vi "Parse Downlink.vi"(7 "CP_DATA IN":u8[](array[numeric]), 8 "error in (no error)":errorcluster, 9 "Parameters":string, 10 "EXID":u32 step=1 format="%06x", 11 "Command":T1) -> (0 "error out":errorcluster, 2 "Downlink":u8[][](array[numeric]) format="%02x")   [LabVIEW 2020]
uses:
  Typedef Command List.ctl
  <vilib>/Utility/miscctls.llb/LVDateTimeRec.ctl
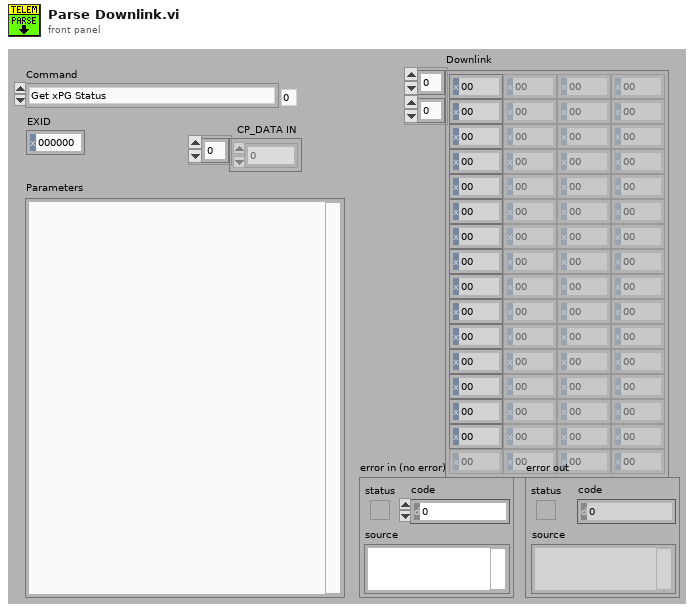
[diagram p1: front panel]
types:
  T1 = typedef "Typedef Command List.ctl" = enum16{"Get xPG Status", "xPG Stimulation", "Select Program", "Increment Program Amplitude", "Decrement Program Amplitude", "Get PoP Constants", "Get PPC Constants", "Get Program Names", "Set Pulse Amplitude", "Increment Pulse Amplitude", "Decrement Pulse Amplitude", "Get Pulse Widths", "Set Pulse Widths", "Increment Pulse Width", "Decrement Pulse Width", "Get Program Frequency", "Set Program Frequency", "Increment Program Frequency", "Decrement Program Frequency", "Inject Event", "Charging Control", "Get xPG Identity", "Set xPG Identity", "Restore Program Defaults", "Get Program Definition", "Set Program Definition", "Get Program Constants", "Set Program Constants", "Get Configurable Device Parameters", "Set Configurable Device Parameters", "Get Pulse Constants", "Set Pulse Constants", "Get Lead Limits", "Set Lead Limits", "Get Channel Calibrations", "Set Channel Calibrations", "<reserved 2>", "<reserved 3>", "<reserved 4>", "<reserved 5>", "<reserved 6>", "<reserved 7>", "Get Stim Asic HV Calibrations", "Set Stim Asic HV Calibrations", "<reserved 8>", "<reserved 9>", "Get CP Data", "Set CP Data", "Clear Log", "Read Log", "Append Log", "Get Patient Program Runtime", "Set Patient Program Runtime", "Impedance Measurement", "Enter Storage Mode", "Echo Short", "Echo Long", "Get General Calibration", "Set General Calibration", "Get Trim List", "Set Trim List", "Get Counter", "Set Counter", "Get Test Stimulation", "Set Test Stimulation", "Get Titration Stimulation", "Set Titration Stimulation", "Get Ramp Time", "Set Ramp Time", "Get VBAT", "Set Software Description Block", "Get Software Description Block", "Write Memory", "Read Memory", "Reset xPG", "Erase Flash Block", "Write Vectors", "Read Vectors", "Diagnostic Data", "Set Background Impedance", "Get Background Impedence ", "Set Test Waveform", "Calibrate Channel", "Get Log Range", "Reserved 0x55", "Reserved 0x56", "MICS Options", "Pair PPC", "Pair POP", "Stop Bootloader", "Tune MICS", "MICS Diagnostics", "Undefined"}
  T2 = enum16{"U8", "U16", "U32", "U64", "I8", "I16", "I32", "I64"}
  T3 = typedef "LVDateTimeRec.ctl" = cluster{"fractional second":dbl, "second":i32, "minute":i32, "hour":i32, "day of month":i32, "month":i32, "year":i32, "day of week":i32, "day of year":i32, "DST":i32}
  T4 = cluster{"CP_DATA IN[0]":u8, "CP_DATA IN[1]":u8, "CP_DATA IN[2]":u8, "CP_DATA IN[3]":u8, "CP_DATA IN[4]":u8, "CP_DATA IN[5]":u8, "CP_DATA IN[6]":u8, "CP_DATA IN[7]":u8, "CP_DATA IN[8]":u8, "CP_DATA IN[9]":u8, "CP_DATA IN[10]":u8, "CP_DATA IN[11]":u8, "CP_DATA IN[12]":u8, "CP_DATA IN[13]":u8, "CP_DATA IN[14]":u8, "CP_DATA IN[15]":u8, "CP_DATA IN[16]":u8, "CP_DATA IN[17]":u8, "CP_DATA IN[18]":u8, "CP_DATA IN[19]":u8, "CP_DATA IN[20]":u8, "CP_DATA IN[21]":u8, "CP_DATA IN[22]":u8, "CP_DATA IN[23]":u8, "CP_DATA IN[24]":u8, "CP_DATA IN[25]":u8, "CP_DATA IN[26]":u8, "CP_DATA IN[27]":u8, "CP_DATA IN[28]":u8, "CP_DATA IN[29]":u8, "CP_DATA IN[30]":u8, "CP_DATA IN[31]":u8, "CP_DATA IN[32]":u8, "CP_DATA IN[33]":u8, "CP_DATA IN[34]":u8, "CP_DATA IN[35]":u8, "CP_DATA IN[36]":u8, "CP_DATA IN[37]":u8, "CP_DATA IN[38]":u8, "CP_DATA IN[39]":u8, "CP_DATA IN[40]":u8, "CP_DATA IN[41]":u8, "CP_DATA IN[42]":u8, "CP_DATA IN[43]":u8, "CP_DATA IN[44]":u8, "CP_DATA IN[45]":u8, "CP_DATA IN[46]":u8, "CP_DATA IN[47]":u8, "CP_DATA IN[48]":u8, "CP_DATA IN[49]":u8, "CP_DATA IN[50]":u8, "CP_DATA IN[51]":u8, "CP_DATA IN[52]":u8, "CP_DATA IN[53]":u8, "CP_DATA IN[54]":u8, "CP_DATA IN[55]":u8, "CP_DATA IN[56]":u8, "CP_DATA IN[57]":u8, "CP_DATA IN[58]":u8, "CP_DATA IN[59]":u8, "CP_DATA IN[60]":u8, "CP_DATA IN[61]":u8, "CP_DATA IN[62]":u8, "CP_DATA IN[63]":u8, "CP_DATA IN[64]":u8, "CP_DATA IN[65]":u8, "CP_DATA IN[66]":u8, "CP_DATA IN[67]":u8, "CP_DATA IN[68]":u8, "CP_DATA IN[69]":u8, "CP_DATA IN[70]":u8, "CP_DATA IN[71]":u8, "CP_DATA IN[72]":u8, "CP_DATA IN[73]":u8, "CP_DATA IN[74]":u8, "CP_DATA IN[75]":u8, "CP_DATA IN[76]":u8, "CP_DATA IN[77]":u8, "CP_DATA IN[78]":u8, "CP_DATA IN[79]":u8, "CP_DATA IN[80]":u8, "CP_DATA IN[81]":u8, "CP_DATA IN[82]":u8, "CP_DATA IN[83]":u8, "CP_DATA IN[84]":u8, "CP_DATA IN[85]":u8, "CP_DATA IN[86]":u8, "CP_DATA IN[87]":u8, "CP_DATA IN[88]":u8, "CP_DATA IN[89]":u8, "CP_DATA IN[90]":u8, "CP_DATA IN[91]":u8, "CP_DATA IN[92]":u8, "CP_DATA IN[93]":u8, "CP_DATA IN[94]":u8, "CP_DATA IN[95]":u8, "CP_DATA IN[96]":u8, "CP_DATA IN[97]":u8, "CP_DATA IN[98]":u8, "CP_DATA IN[99]":u8, "CP_DATA IN[100]":u8, "CP_DATA IN[101]":u8, "CP_DATA IN[102]":u8, "CP_DATA IN[103]":u8, "CP_DATA IN[104]":u8, "CP_DATA IN[105]":u8, "CP_DATA IN[106]":u8, "CP_DATA IN[107]":u8, "CP_DATA IN[108]":u8, "CP_DATA IN[109]":u8, "CP_DATA IN[110]":u8, "CP_DATA IN[111]":u8, "CP_DATA IN[112]":u8, "CP_DATA IN[113]":u8, "CP_DATA IN[114]":u8, "CP_DATA IN[115]":u8, "CP_DATA IN[116]":u8, "CP_DATA IN[117]":u8, "CP_DATA IN[118]":u8, "CP_DATA IN[119]":u8, "CP_DATA IN[120]":u8, "CP_DATA IN[121]":u8, "CP_DATA IN[122]":u8, "CP_DATA IN[123]":u8, "CP_DATA IN[124]":u8, "CP_DATA IN[125]":u8, "CP_DATA IN[126]":u8, "CP_DATA IN[127]":u8, "CP_DATA IN[128]":u8, "CP_DATA IN[129]":u8, "CP_DATA IN[130]":u8, "CP_DATA IN[131]":u8, "CP_DATA IN[132]":u8, "CP_DATA IN[133]":u8, "CP_DATA IN[134]":u8, "CP_DATA IN[135]":u8, "CP_DATA IN[136]":u8, "CP_DATA IN[137]":u8, "CP_DATA IN[138]":u8, "CP_DATA IN[139]":u8, "CP_DATA IN[140]":u8, "CP_DATA IN[141]":u8, "CP_DATA IN[142]":u8, "CP_DATA IN[143]":u8, "CP_DATA IN[144]":u8, "CP_DATA IN[145]":u8, "CP_DATA IN[146]":u8, "CP_DATA IN[147]":u8, "CP_DATA IN[148]":u8, "CP_DATA IN[149]":u8, "CP_DATA IN[150]":u8, "CP_DATA IN[151]":u8, "CP_DATA IN[152]":u8, "CP_DATA IN[153]":u8, "CP_DATA IN[154]":u8, "CP_DATA IN[155]":u8, "CP_DATA IN[156]":u8, "CP_DATA IN[157]":u8, "CP_DATA IN[158]":u8, "CP_DATA IN[159]":u8, "CP_DATA IN[160]":u8, "CP_DATA IN[161]":u8, "CP_DATA IN[162]":u8, "CP_DATA IN[163]":u8, "CP_DATA IN[164]":u8, "CP_DATA IN[165]":u8, "CP_DATA IN[166]":u8, "CP_DATA IN[167]":u8, "CP_DATA IN[168]":u8, "CP_DATA IN[169]":u8, "CP_DATA IN[170]":u8, "CP_DATA IN[171]":u8, "CP_DATA IN[172]":u8, "CP_DATA IN[173]":u8, "CP_DATA IN[174]":u8, "CP_DATA IN[175]":u8, "CP_DATA IN[176]":u8, "CP_DATA IN[177]":u8, "CP_DATA IN[178]":u8, "CP_DATA IN[179]":u8, "CP_DATA IN[180]":u8, "CP_DATA IN[181]":u8, "CP_DATA IN[182]":u8, "CP_DATA IN[183]":u8, "CP_DATA IN[184]":u8, "CP_DATA IN[185]":u8, "CP_DATA IN[186]":u8, "CP_DATA IN[187]":u8, "CP_DATA IN[188]":u8, "CP_DATA IN[189]":u8, "CP_DATA IN[190]":u8, "CP_DATA IN[191]":u8, "CP_DATA IN[192]":u8, "CP_DATA IN[193]":u8, "CP_DATA IN[194]":u8, "CP_DATA IN[195]":u8, "CP_DATA IN[196]":u8, "CP_DATA IN[197]":u8, "CP_DATA IN[198]":u8, "CP_DATA IN[199]":u8, "CP_DATA IN[200]":u8, "CP_DATA IN[201]":u8, "CP_DATA IN[202]":u8, "CP_DATA IN[203]":u8, "CP_DATA IN[204]":u8, "CP_DATA IN[205]":u8, "CP_DATA IN[206]":u8, "CP_DATA IN[207]":u8, "CP_DATA IN[208]":u8, "CP_DATA IN[209]":u8, "CP_DATA IN[210]":u8, "CP_DATA IN[211]":u8, "CP_DATA IN[212]":u8, "CP_DATA IN[213]":u8, "CP_DATA IN[214]":u8, "CP_DATA IN[215]":u8, "CP_DATA IN[216]":u8, "CP_DATA IN[217]":u8, "CP_DATA IN[218]":u8, "CP_DATA IN[219]":u8, "CP_DATA IN[220]":u8, "CP_DATA IN[221]":u8, "CP_DATA IN[222]":u8, "CP_DATA IN[223]":u8, "CP_DATA IN[224]":u8, "CP_DATA IN[225]":u8, "CP_DATA IN[226]":u8, "CP_DATA IN[227]":u8, "CP_DATA IN[228]":u8, "CP_DATA IN[229]":u8, "CP_DATA IN[230]":u8, "CP_DATA IN[231]":u8, "CP_DATA IN[232]":u8, "CP_DATA IN[233]":u8, "CP_DATA IN[234]":u8, "CP_DATA IN[235]":u8, "CP_DATA IN[236]":u8, "CP_DATA IN[237]":u8, "CP_DATA IN[238]":u8, "CP_DATA IN[239]":u8, "CP_DATA IN[240]":u8, "CP_DATA IN[241]":u8, "CP_DATA IN[242]":u8, "CP_DATA IN[243]":u8, "CP_DATA IN[244]":u8, "CP_DATA IN[245]":u8, "CP_DATA IN[246]":u8, "CP_DATA IN[247]":u8, "CP_DATA IN[248]":u8, "CP_DATA IN[249]":u8, "CP_DATA IN[250]":u8, "CP_DATA IN[251]":u8, "CP_DATA IN[252]":u8, "CP_DATA IN[253]":u8, "CP_DATA IN[254]":u8, "CP_DATA IN[255]":u8}
  T5 = cluster{"DATA[0]":u8, "DATA[1]":u8, "DATA[2]":u8, "DATA[3]":u8, "DATA[4]":u8, "DATA[5]":u8, "DATA[6]":u8, "DATA[7]":u8, "DATA[8]":u8, "DATA[9]":u8, "DATA[10]":u8, "DATA[11]":u8, "DATA[12]":u8, "DATA[13]":u8, "DATA[14]":u8}
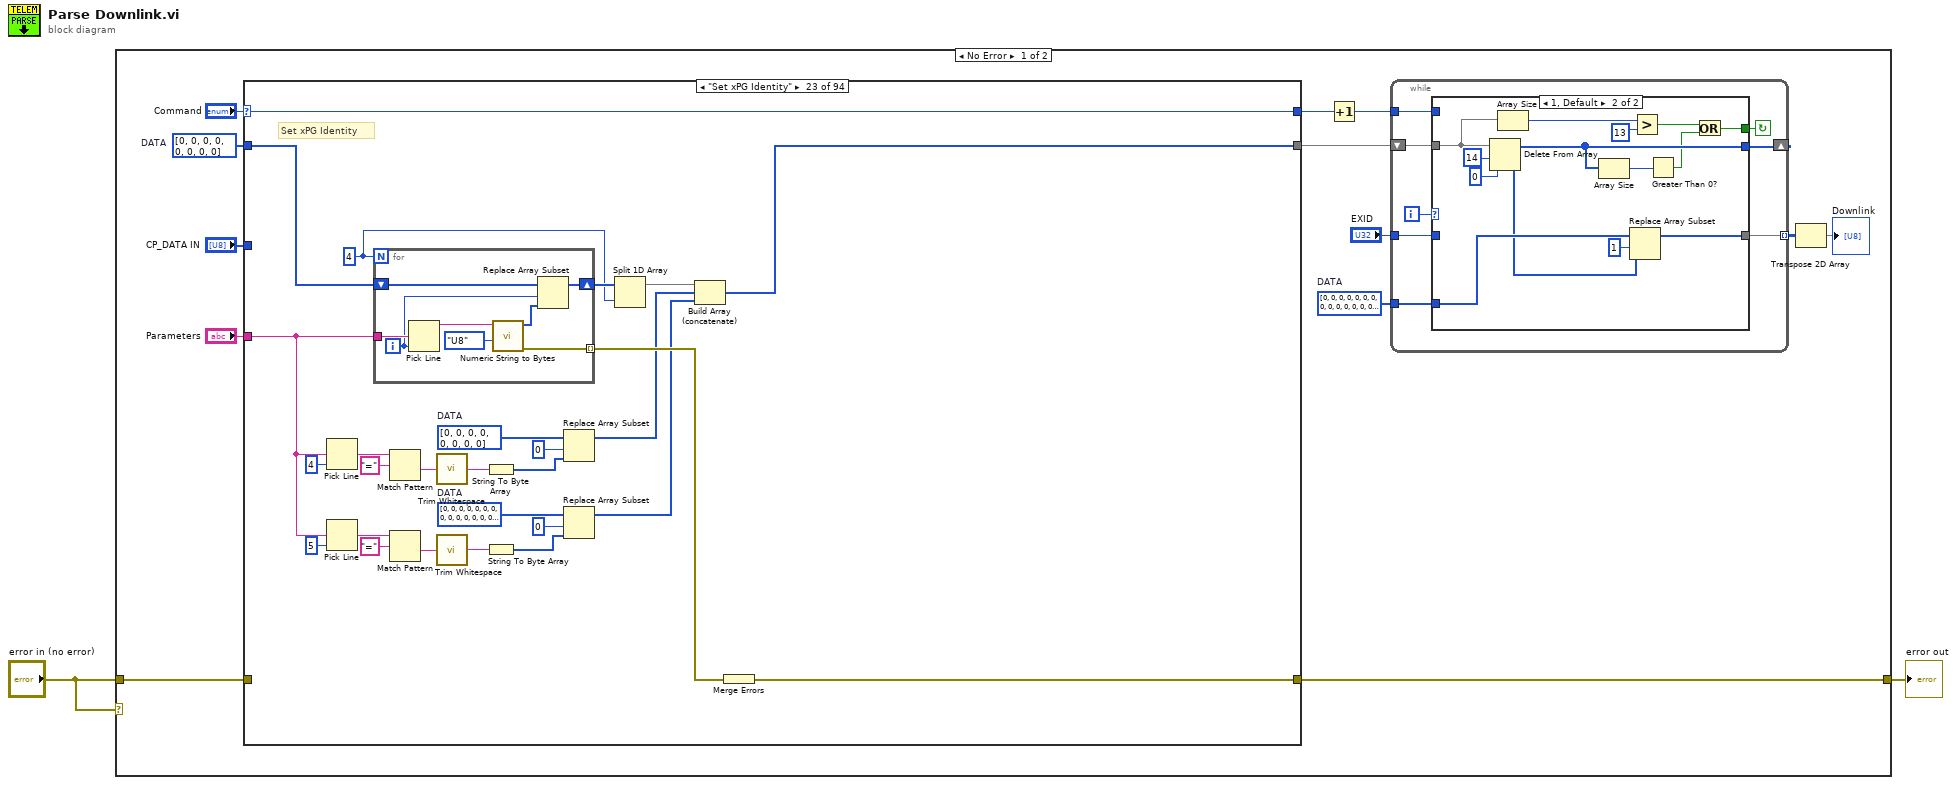
[diagram p0: block diagram]
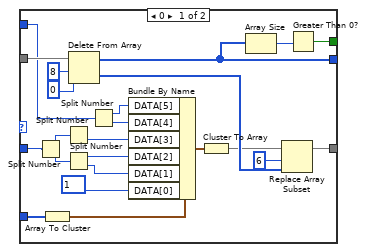
[diagram p2: hidden frame]
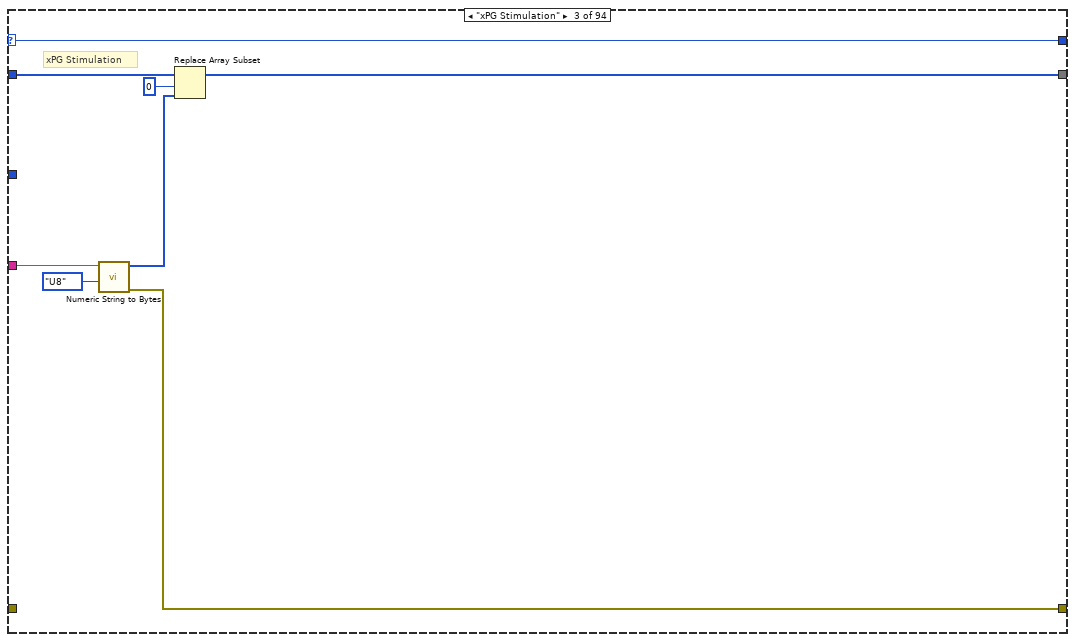
[diagram p5: hidden frame]
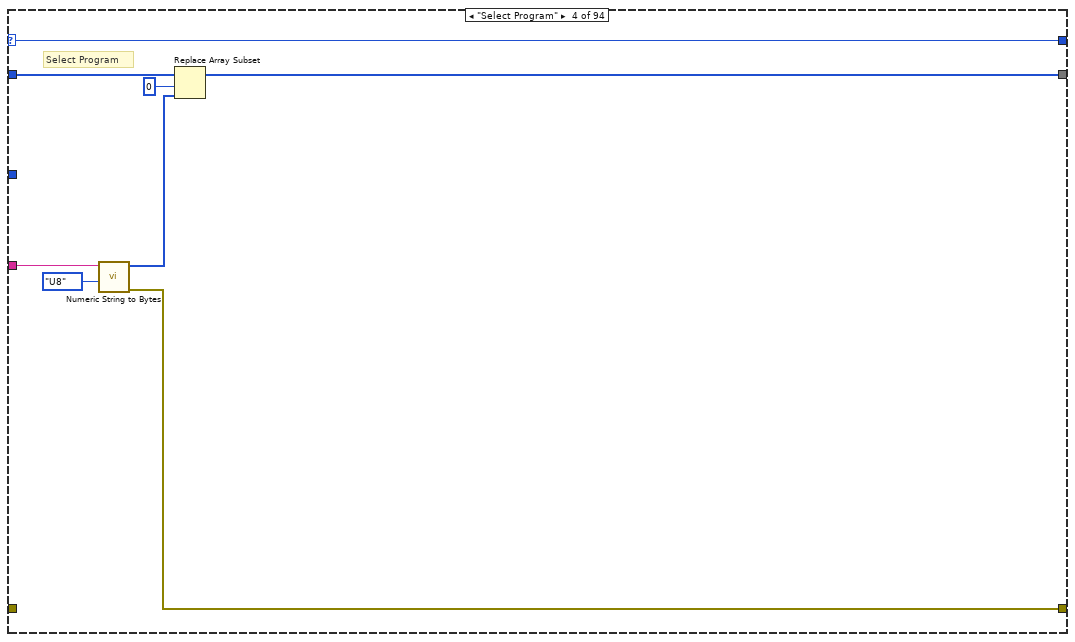
[diagram p6: hidden frame]
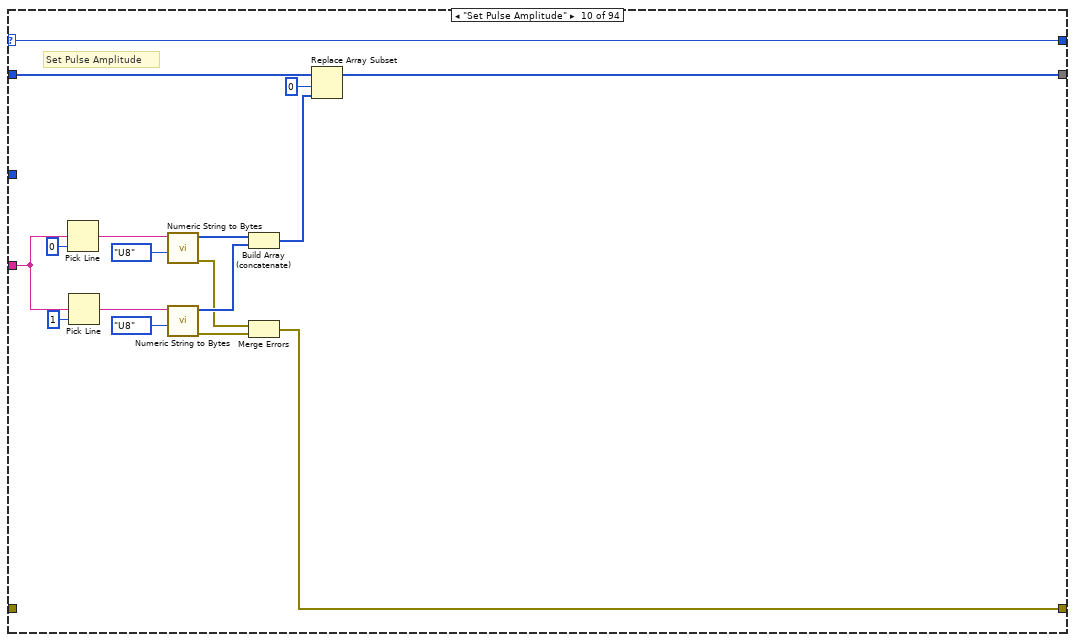
[diagram p12: hidden frame]
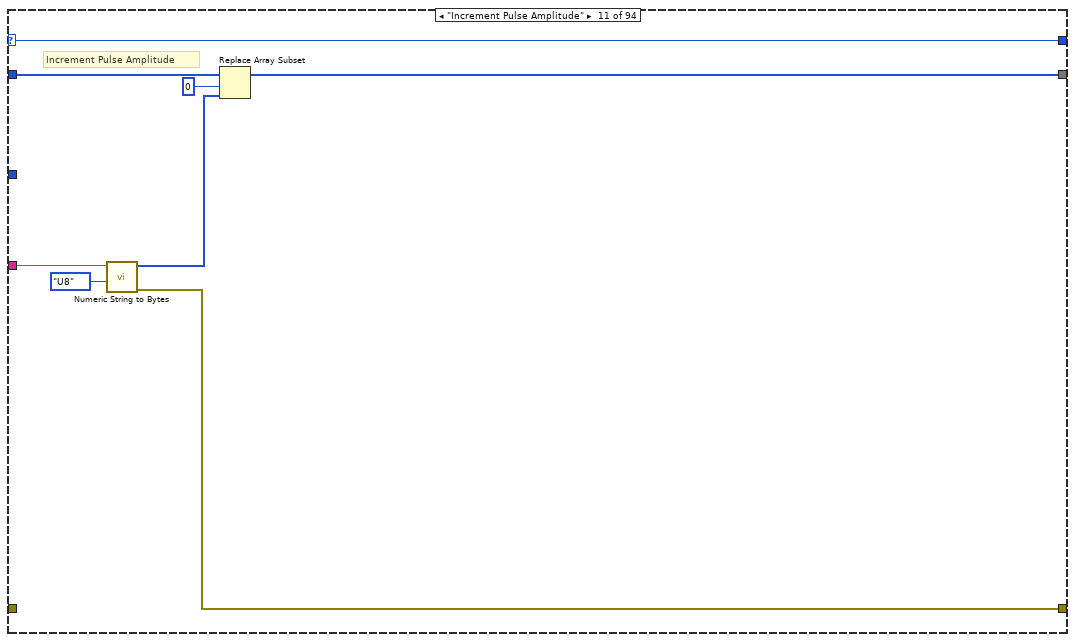
[diagram p13: hidden frame]
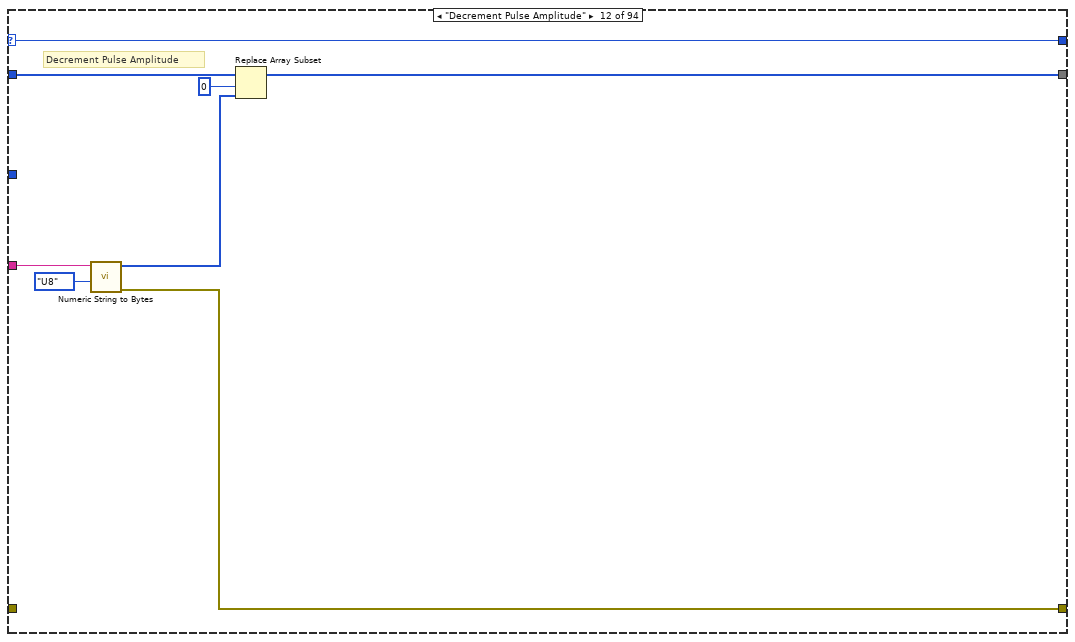
[diagram p14: hidden frame]
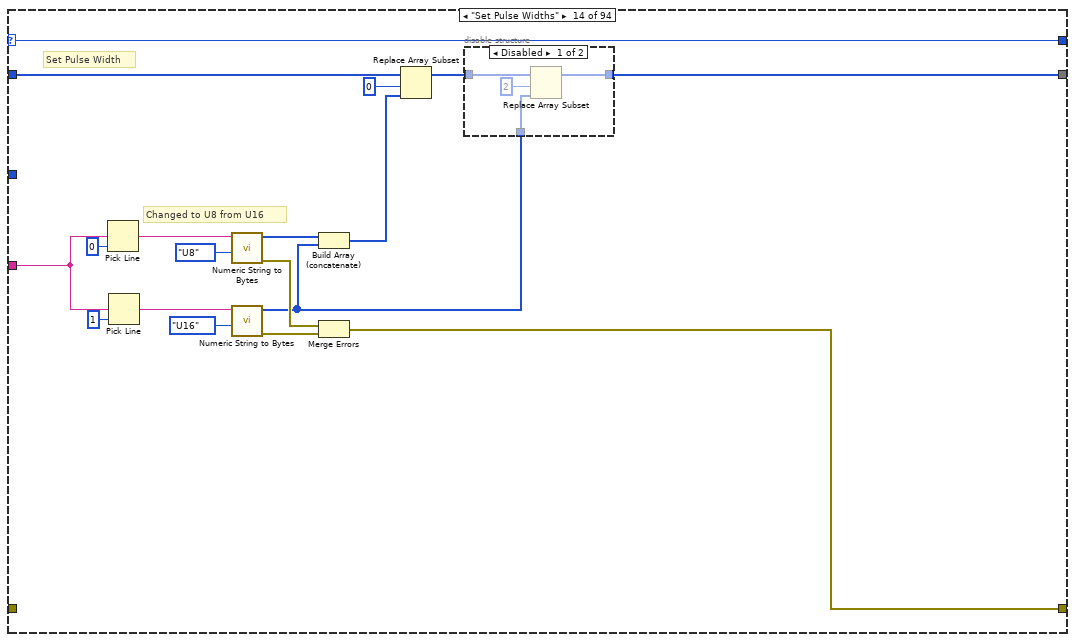
[diagram p16: hidden frame]
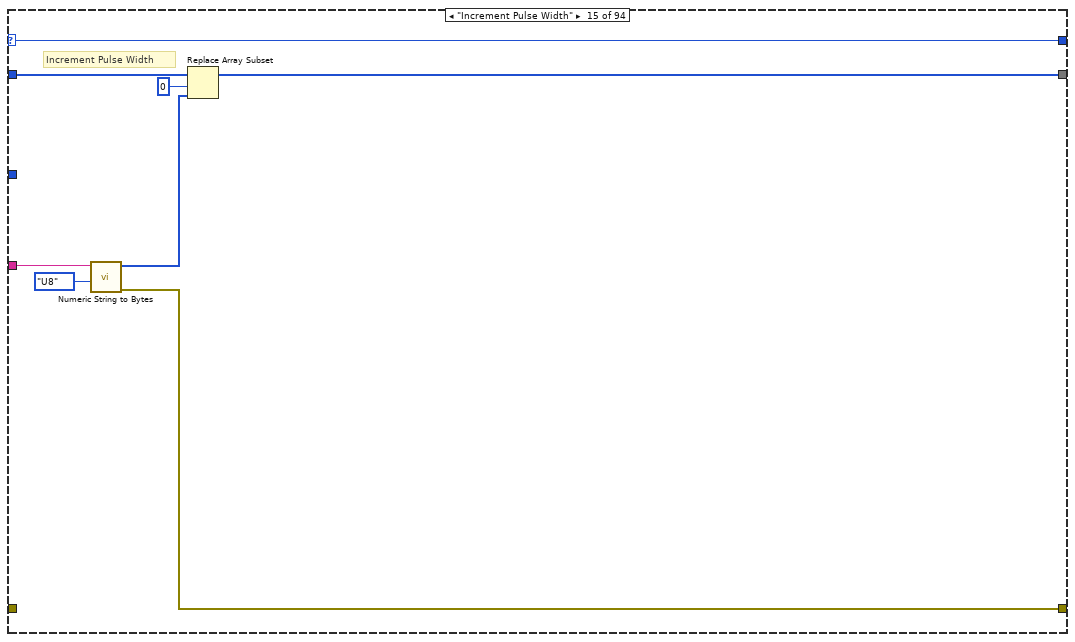
[diagram p18: hidden frame]
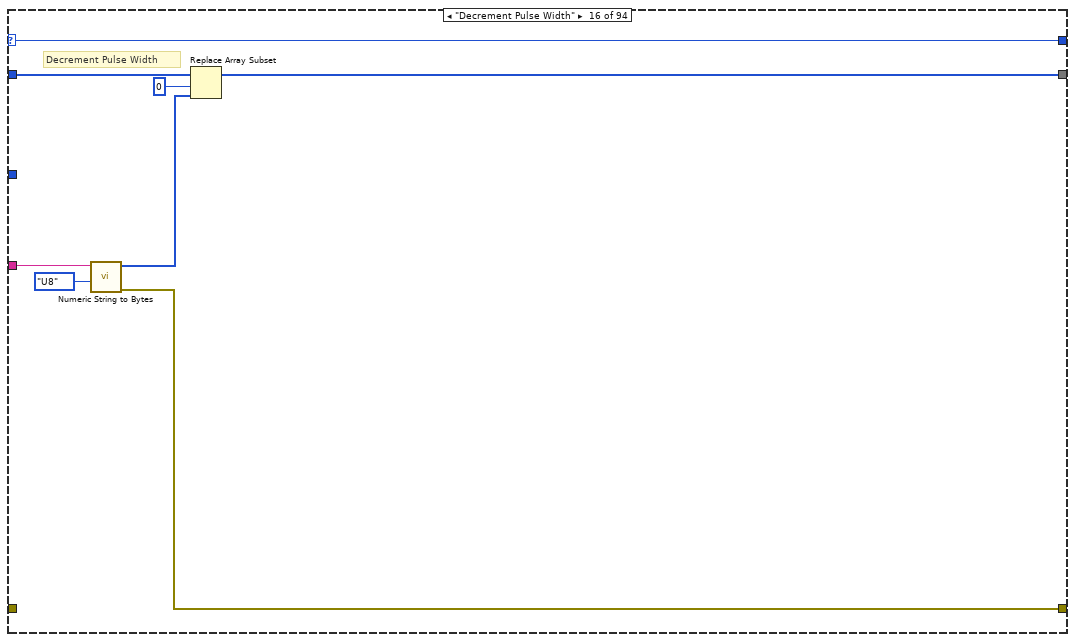
[diagram p19: hidden frame]
diagram:
  n1 = case shown="No Error" "error in (no error)" {
    tunnel: "error in (no error)" -> [w8 w1324]
    tunnel: [w7 w1324] -> w2
    frame No Error {
      w9 = u8[] [0, 0, 0, 0, 0, 0, 0, 0]  # DATA
      w10 = u8[] [0, 0, 0, 0, 0, 0, 0, 0, 0, 0, 0, 0, 0, 0, 0]  # DATA
      n2 = case shown="\"Set xPG Identity\"" "Command" {
        selector: "Command" -> [w63 w66 w74 w82 w85 w88 w91 w94 w97 w114 w122 w130 w133 w151 w164 w172 w175 w183 w186 w189 w192 w195 w222 w238 w246 w253 w396 w410 w423 w498 w516 w535 w546 w553 w569 w582 w594 w601 w617 w629 w637 w656 w694 w702 w720 w743 w746 w752 w758 w761 w767 w869 w871 w961 w980 w983 w1007 w1064 w1083 w1115 w1123 w1126 w1129 w1132 w1154 w1171 w1174 w1177 w1180 w1183 w1200 w1214 w1228 w1231 w1233 w1236 w1247 w1249 w1252 w1255 w1258 w1261 w1264 w1267 w1296 w1298 w1301 w1304 w1307 w1310 w1313 w1316 w1319 w1322]
        tunnel: "Parameters" -> [_ _ w72 w80 _ _ _ _ _ w113 w120 w128 _ w139 w162 w170 _ w181 _ _ _ _ w221 w236 w244 w248 _ w398 _ w428 _ w522 _ w550 w564 w571 _ w598 w615 w624 w635 w640 w659 w700 w703 w721 _ _ _ _ w763 w864 w873 w959 w964 _ w989 _ w1074 _ w1120 _ _ _ w1143 w1166 _ _ _ _ w1196 w1204 w1218 _ _ _ w1245 _ _ _ _ _ _ _ w1287 _ _ _ _ _ _ _ _ _]
        tunnel: [w63 w66 w74 w82 w85 w88 w91 w94 w97 w114 w122 w130 w133 w151 w164 w172 w175 w183 w186 w189 w192 w195 w222 w238 w246 w253 w396 w410 w423 w498 w516 w535 w546 w553 w569 w582 w594 w601 w617 w629 w637 w656 w694 w702 w720 w743 w746 w752 w758 w761 w767 w869 w871 w961 w980 w983 w1007 w1064 w1083 w1115 w1123 w1126 w1129 w1132 w1154 w1171 w1174 w1177 w1180 w1183 w1200 w1214 w1228 w1231 w1233 w1236 w1247 w1249 w1252 w1255 w1258 w1261 w1264 w1267 w1296 w1298 w1301 w1304 w1307 w1310 w1313 w1316 w1319 w1322] -> w15
        tunnel: [w62 w65 w70 w78 w84 w87 w90 w93 w96 w106 w118 w126 w132 w137 w160 w168 w174 w179 w185 w188 w191 w194 w201 w234 w242 w249 w395 w408 w422 w495 w515 w532 w545 w548 w562 w574 w593 w596 w613 w623 w633 w654 w692 w698 w718 w741 w745 w748 w754 w760 w764 w862 w872 w957 w978 w981 w986 w1062 w1069 w1113 w1117 w1124 w1127 w1130 w1142 w1155 w1172 w1175 w1178 w1181 w1184 w1209 w1223 w1230 w1232 w1235 w1239 w1248 w1251 w1254 w1257 w1260 w1263 w1266 w1271 w1297 w1300 w1303 w1306 w1309 w1312 w1315 w1318 w1321] -> w13
        tunnel: w9 -> [w62 w65 w73 w81 w84 w87 w90 w93 w96 w105 w121 w129 w132 w144 w163 w171 w174 w182 w185 w188 w191 w194 w212 w237 w245 _ w395 _ w422 _ w515 _ w545 _ w563 _ w593 _ w616 _ w636 w655 w693 w701 w719 w742 w745 _ _ w760 _ w865 _ w960 w979 w981 _ w1062 _ w1113 w1119 w1124 w1127 w1130 _ w1156 w1172 w1175 w1178 w1181 w1187 _ _ w1230 w1232 w1235 w1241 w1248 w1251 w1254 w1257 w1260 w1263 w1266 w1272 w1297 w1300 w1303 w1306 w1309 w1312 w1315 w1318 w1321]
        tunnel: w8 -> [w61 w64 _ _ w83 w86 w89 w92 w95 _ _ _ w131 _ _ _ w173 _ w184 w187 w190 w193 _ _ _ w251 w394 _ w421 _ w514 _ w544 _ _ _ w592 _ _ _ _ _ _ _ _ _ w744 w747 w753 w759 _ _ _ _ _ w982 _ w1063 _ w1114 _ w1125 w1128 w1131 _ _ w1173 w1176 w1179 w1182 _ _ _ w1229 w1234 w1237 _ w1250 w1253 w1256 w1259 w1262 w1265 w1268 _ w1299 w1302 w1305 w1308 w1311 w1314 w1317 w1320 w1323]
        tunnel: [w61 w64 w71 w79 w83 w86 w89 w92 w95 w98 w119 w127 w131 w140 w161 w169 w173 w180 w184 w187 w190 w193 w202 w235 w243 w250 w394 w401 w421 w496 w514 w531 w544 w551 w565 w580 w592 w599 w614 w628 w634 w641 w678 w699 w704 w727 w744 w747 w753 w759 w765 w863 w870 w958 w965 w982 w987 w1063 w1065 w1114 w1116 w1125 w1128 w1131 w1141 w1157 w1173 w1176 w1179 w1182 w1188 w1201 w1215 w1229 w1234 w1237 w1238 w1250 w1253 w1256 w1259 w1262 w1265 w1268 w1274 w1299 w1302 w1305 w1308 w1311 w1314 w1317 w1320 w1323] -> w7
        tunnel: "CP_DATA IN" -> [_ _ _ _ _ _ _ _ _ _ _ _ _ _ _ _ _ _ _ _ _ _ _ _ _ _ _ _ _ _ _ _ _ _ _ _ _ _ _ w620 _ _ _ _ _ _ _ w751 w757 _ _ _ _ _ _ _ _ _ _ _ _ _ _ _ w1134 _ _ _ _ _ _ _ _ _ _ _ _ _ _ _ _ _ _ _ _ _ _ _ _ _ _ _ _ _]
        frame Default {
          # "NULL"
        }
        frame "Get xPG Status" {
          # "Get xPG Status"
        }
        frame "xPG Stimulation" {
          # "xPG Stimulation"
          n3 = call "Numeric String to Bytes.vi"("Type"=T2."U8", "String"=w72) -> ("error out"=w71:errorcluster, "Byte Data"=w68:u8[])  [unwired: 8 in]
          n4 = Replace Array Subset(array=w73, new element=w68, index=0) -> (w70:u8[])
        }
        frame "Select Program" {
          # "Select Program"
          n5 = call "Numeric String to Bytes.vi"("Type"=T2."U8", "String"=w80) -> ("error out"=w79:errorcluster, "Byte Data"=w76:u8[])  [unwired: 8 in]
          n6 = Replace Array Subset(array=w81, new element=w76, index=0) -> (w78:u8[])
        }
        frame "Increment Program Amplitude" {
          # "Increment Program Amplitude"
        }
        frame "Decrement Program Amplitude" {
          # "Decrement Program Amplitude"
        }
        frame "Get PoP Constants" {
          # "Get PoP Constants"
        }
        frame "Get PPC Constants" {
          # "Get PPC Constants"
        }
        frame "Get Program Names" {
          # "Get Program Names"
        }
        frame "Set Pulse Amplitude" {
          # "Set Pulse Amplitude"
          n7 = Pick Line(multi-line string=w113, line index=0) -> (output string=w107:string)  [unwired: 1 in]
          n8 = Pick Line(multi-line string=w113, line index=1) -> (output string=w108:string)  [unwired: 1 in]
          n9 = call "Numeric String to Bytes.vi"("Type"=T2."U8", "String"=w107) -> ("error out"=w100:errorcluster, "Byte Data"=w104:u8[])  [unwired: 8 in]
          n10 = call "Numeric String to Bytes.vi"("Type"=T2."U8", "String"=w108) -> ("error out"=w99:errorcluster, "Byte Data"=w103:u8[])  [unwired: 8 in]
          n11 = Build Array (concatenate)(w104, w103) -> (w101:u8[])
          n12 = Merge Errors(w100, w99) -> (w98:errorcluster)
          n13 = Replace Array Subset(array=w105, new element=w101, index=0) -> (w106:u8[])
        }
        frame "Increment Pulse Amplitude" {
          # "Increment Pulse Amplitude"
          n14 = call "Numeric String to Bytes.vi"("Type"=T2."U8", "String"=w120) -> ("error out"=w119:errorcluster, "Byte Data"=w116:u8[])  [unwired: 8 in]
          n15 = Replace Array Subset(array=w121, new element=w116, index=0) -> (w118:u8[])
        }
        frame "Decrement Pulse Amplitude" {
          # "Decrement Pulse Amplitude"
          n16 = call "Numeric String to Bytes.vi"("Type"=T2."U8", "String"=w128) -> ("error out"=w127:errorcluster, "Byte Data"=w124:u8[])  [unwired: 8 in]
          n17 = Replace Array Subset(array=w129, new element=w124, index=0) -> (w126:u8[])
        }
        frame "Get Pulse Widths" {
          # "Get Pulse Widths"
        }
        frame "Set Pulse Widths" {
          # "Changed to U8 from U16"
          # "Set Pulse Width"
          n18 = Pick Line(multi-line string=w139, line index=0) -> (output string=w145:string)  [unwired: 1 in]
          n19 = Pick Line(multi-line string=w139, line index=1) -> (output string=w146:string)  [unwired: 1 in]
          n20 = call "Numeric String to Bytes.vi"("Type"=T2."U8", "String"=w145) -> ("error out"=w142:errorcluster, "Byte Data"=w136:u8[])  [unwired: 8 in]
          n21 = call "Numeric String to Bytes.vi"("Type"=T2."U16", "String"=w146) -> ("error out"=w141:errorcluster, "Byte Data"=w135:u8[])  [unwired: 8 in]
          n22 = Build Array (concatenate)(w136, w135) -> (w134:u8[])
          n23 = Merge Errors(w142, w141) -> (w140:errorcluster)
          n24 = Replace Array Subset(array=w144, new element=w134, index=0) -> (w138:u8[])
          n25 = disable-structure shown="Disabled" {
            disable-tunnel: w135 -> [w154 _]
            disable-tunnel: w138 -> [w153 w156]
            disable-tunnel: [w152 w156] -> w137
            frame Disabled {
              n26 = Replace Array Subset(array=w153, new element=w154, index=2) -> (w152:u8[])
            }
            frame Enabled {
            }
          }
        }
        frame "Increment Pulse Width" {
          # "Increment Pulse Width"
          n27 = call "Numeric String to Bytes.vi"("Type"=T2."U8", "String"=w162) -> ("error out"=w161:errorcluster, "Byte Data"=w158:u8[])  [unwired: 8 in]
          n28 = Replace Array Subset(array=w163, new element=w158, index=0) -> (w160:u8[])
        }
        frame "Decrement Pulse Width" {
          # "Decrement Pulse Width"
          n29 = call "Numeric String to Bytes.vi"("Type"=T2."U8", "String"=w170) -> ("error out"=w169:errorcluster, "Byte Data"=w166:u8[])  [unwired: 8 in]
          n30 = Replace Array Subset(array=w171, new element=w166, index=0) -> (w168:u8[])
        }
        frame "Get Program Frequency" {
          # "Get Program Frequency"
        }
        frame "Set Program Frequency" {
          # "Set Program Frequency"
          n31 = call "Numeric String to Bytes.vi"("Type"=T2."U8", "String"=w181) -> ("error out"=w180:errorcluster, "Byte Data"=w177:u8[])  [unwired: 8 in]
          n32 = Replace Array Subset(array=w182, new element=w177, index=0) -> (w179:u8[])
        }
        frame "Increment Program Frequency" {
          # "Increment Program Frequency"
        }
        frame "Decrement Program Frequency" {
          # "Decrement Program Frequency"
        }
        frame "Charging Control" {
          # "Charging Control"
        }
        frame "Get xPG Identity" {
          # "Get xPG Identity"
        }
        frame "Set xPG Identity" {
          w215 = u8[] [0, 0, 0, 0, 0, 0, 0, 0, 0, 0, 0, 0, 0, 0, 0, 0]  # DATA
          w216 = u8[] [0, 0, 0, 0, 0, 0, 0, 0]  # DATA
          w199 = 4
          # "Set xPG Identity"
          n33 = Pick Line(multi-line string=w221, line index=4) -> (output string=w208:string)  [unwired: 1 in]
          n34 = Pick Line(multi-line string=w221, line index=5) -> (output string=w205:string)  [unwired: 1 in]
          n35 = for {
            N: w199 -> [_]
            tunnel: w221 -> [w230]
            shift-right: [w225] -> w200
            shift-left: w212 -> [w226]
            tunnel: [w227] -> w203 mode=indexing
            i -> [w223]
            n36 = Pick Line(multi-line string=w230, line index=w223) -> (output string=w229:string)  [unwired: 1 in]
            n37 = call "Numeric String to Bytes.vi"("Type"=T2."U8", "String"=w229) -> ("error out"=w227:errorcluster, "Byte Data"=w224:u8[])  [unwired: 8 in]
            n38 = Replace Array Subset(array=w226, new element=w224, index=w223) -> (w225:u8[])
          }
          n39 = Match Pattern(string=w208, regular expression="=") -> (after substring=w207:string)  [unwired: 1 in, 3 out]
          n40 = Match Pattern(string=w205, regular expression="=") -> (after substring=w204:string)  [unwired: 1 in, 3 out]
          n41 = call <vilib>:"Trim Whitespace.vi"("string"=w207) -> ("trimmed string"=w218:string)  [unwired: 1 in]
          n42 = call <vilib>:"Trim Whitespace.vi"("string"=w204) -> ("trimmed string"=w217:string)  [unwired: 1 in]
          n43 = String To Byte Array(string=w218) -> (unsigned byte array=w213:u8[])
          n44 = String To Byte Array(string=w217) -> (unsigned byte array=w214:u8[])
          n45 = Replace Array Subset(array=w216, new element=w213, index=0) -> (w197:u8[])
          n46 = Replace Array Subset(array=w215, new element=w214, index=0) -> (w196:u8[])
          n47 = Split 1D Array(array=w200, index=w199) -> (first subarray=w198:u8[])  [unwired: 1 out]
          n48 = Build Array (concatenate)(w198, w197, w196) -> (w201:u8[])
          n49 = Merge Errors(w203) -> (w202:errorcluster)
        }
        frame "Restore Program Defaults" {
          # "Restore Program Defaults"
          n50 = call "Numeric String to Bytes.vi"("Type"=T2."U16", "String"=w236) -> ("error out"=w235:errorcluster, "Byte Data"=w232:u8[])  [unwired: 8 in]
          n51 = Replace Array Subset(array=w237, new element=w232, index=0) -> (w234:u8[])
        }
        frame "Get Program Definition" {
          # "Get Program Definition"
          n52 = call "Numeric String to Bytes.vi"("Type"=T2."U8", "String"=w244) -> ("error out"=w243:errorcluster, "Byte Data"=w240:u8[])  [unwired: 8 in]
          n53 = Replace Array Subset(array=w245, new element=w240, index=0) -> (w242:u8[])
        }
        frame "Set Program Definition" {
          w252 = u8[] []  # DATA
          # "Set Program Definition"
          n54 = while {
            shift-right: [w257] -> w249
            shift-left: w252 -> [w258]
            shift-right: [w263] -> w250
            shift-left: w251 -> [w264]
            tunnel: w248 -> [w256]
            shift-right: [w254] -> _
            shift-left: 0 -> [w255]
            i -> [w259]
            stop <- w260 stop-if-true
            n55 = case shown="0" w259 {
              tunnel: w264 -> [w276 w328]
              tunnel: [w275 w327] -> w263
              tunnel: [FALSE ("status") TRUE ("status")] -> w261
              tunnel: w258 -> [w289 w331]
              tunnel: [w288 w330] -> w257
              tunnel: w256 -> [w291 w325]
              tunnel: w255 -> [_ w326]
              tunnel: [14 ("line index") w323] -> w254
              frame 0 {
                w305 = u8[] [0, 0, 0, 0, 0, 0, 0, 0, 0, 0, 0, 0, 0, 0, 0, 0]  # DATA
                # "Changed to U8 from U16"
                n56 = Pick Line(multi-line string=w291, line index=3) -> (output string=w272:string)  [unwired: 1 in]
                n57 = Pick Line(multi-line string=w291, line index=0) -> (output string=w298:string)  [unwired: 1 in]
                n58 = Pick Line(multi-line string=w291, line index=1) -> (output string=w299:string)  [unwired: 1 in]
                n59 = Pick Line(multi-line string=w291, line index=2) -> (output string=w300:string)  [unwired: 1 in]
                n60 = Pick Line(multi-line string=w291, line index=12) -> (output string=w295:string)  [unwired: 1 in]
                n61 = Pick Line(multi-line string=w291, line index=13) -> (output string=w292:string)  [unwired: 1 in]
                n62 = for {
                  N: 8 -> [_]
                  tunnel: w291 -> [w322]
                  shift-right: [w314] -> w285
                  shift-left: w289 -> [w315]
                  tunnel: [w313] -> w270 mode=indexing
                  i -> [w320]
                  n63 = Add(x=4 ("line index"), y=w320) -> (x+y=w319:i32)
                  n64 = Pick Line(multi-line string=w322, line index=w319) -> (output string=w317:string)  [unwired: 1 in]
                  n65 = call "Numeric String to Bytes.vi"("Type"=T2."U8", "String"=w317) -> ("error out"=w313:errorcluster, "Byte Data"=w316:u8[])  [unwired: 8 in]
                  n66 = Build Array (concatenate)(w315, w316) -> (w314:u8[])
                }
                n67 = Match Pattern(string=w272, regular expression="=") -> (after substring=w271:string)  [unwired: 1 in, 3 out]
                n68 = call <vilib>:"Trim Whitespace.vi"("string"=w271) -> ("trimmed string"=w308:string)  [unwired: 1 in]
                n69 = call "Numeric String to Bytes.vi"("Type"=T2."U8", "String"=w298) -> ("error out"=w281:errorcluster, "Byte Data"=w287:u8[])  [unwired: 8 in]
                n70 = call "Numeric String to Bytes.vi"("Type"=T2."U8", "String"=w299) -> ("error out"=w280:errorcluster, "Byte Data"=w269:u8[])  [unwired: 8 in]
                n71 = call "Numeric String to Bytes.vi"("Type"=T2."U8", "String"=w300) -> ("error out"=w279:errorcluster, "Byte Data"=w286:u8[])  [unwired: 8 in]
                n72 = call "Numeric String to Bytes.vi"("Type"=T2."U8", "String"=w295) -> ("error out"=w278:errorcluster, "Byte Data"=w284:u8[])  [unwired: 8 in]
                n73 = call "Numeric String to Bytes.vi"("Type"=T2."U8", "String"=w292) -> ("error out"=w277:errorcluster, "Byte Data"=w283:u8[])  [unwired: 8 in]
                n74 = String To Byte Array(string=w308) -> (unsigned byte array=w307:u8[])
                n75 = Replace Array Subset(array=w305, new element=w307, index=0) -> (w265:u8[])
                n76 = Split 1D Array(array=w265, index=16) -> (first subarray=w266:u8[])  [unwired: 1 out]
                n77 = Build Array (concatenate)(w289, w287, u8[] [0] ("array"), w269, w286, w266, w285, w284, w283) -> (w288:u8[])
                n78 = Build Array (concatenate)(w281, w280, w279, w270, w278, w277, w276) -> (w274:errorcluster[])
                n79 = Merge Errors(w274) -> (w275:errorcluster)
              }
              frame 1, Default {
                n80 = for {
                  N: 4 -> [_]
                  shift-right: [w349] -> w330
                  shift-left: w331 -> [w366]
                  shift-right: [w351] -> w327
                  shift-left: w328 -> [w358]
                  tunnel: w325 -> [w343]
                  shift-right: [w337] -> w323
                  shift-left: w326 -> [w344]
                  w342 = u8[] []  # DATA
                  w335 = u8[] [0, 0, 0, 0, 0, 0, 0, 0, 0, 0, 0, 0, 0, 0, 0, 0]  # DATA
                  n81 = Increment(x=w344) -> (x+1=w338:i32)
                  n82 = Increment(x=w338) -> (x+1=w369:i32)
                  n83 = Pick Line(multi-line string=w343, line index=w344) -> (output string=w341:string)  [unwired: 1 in]
                  n84 = Pick Line(multi-line string=w343, line index=w338) -> (output string=w381:string)  [unwired: 1 in]
                  n85 = Increment(x=w369) -> (x+1=w370:i32)
                  n86 = Pick Line(multi-line string=w343, line index=w369) -> (output string=w382:string)  [unwired: 1 in]
                  n87 = Match Pattern(string=w341, regular expression="=") -> (after substring=w340:string)  [unwired: 1 in, 3 out]
                  n88 = Increment(x=w370) -> (x+1=w371:i32)
                  n89 = Pick Line(multi-line string=w343, line index=w370) -> (output string=w375:string)  [unwired: 1 in]
                  n90 = Increment(x=w371) -> (x+1=w372:i32)
                  n91 = Pick Line(multi-line string=w343, line index=w371) -> (output string=w376:string)  [unwired: 1 in]
                  n92 = call <vilib>:"Trim Whitespace.vi"("string"=w340) -> ("trimmed string"=w347:string)  [unwired: 1 in]
                  n93 = Increment(x=w372) -> (x+1=w368:i32)
                  n94 = Pick Line(multi-line string=w343, line index=w372) -> (output string=w377:string)  [unwired: 1 in]
                  n95 = Increment(x=w368) -> (x+1=w367:i32)
                  n96 = String To Byte Array(string=w347) -> (unsigned byte array=w346:u8[])
                  n97 = Pick Line(multi-line string=w343, line index=w368) -> (output string=w373:string)  [unwired: 1 in]
                  n98 = for {
                    N: 26 -> [_]
                    tunnel: w343 -> [w393]
                    shift-right: [w388] -> w359
                    shift-left: w342 -> [w389]
                    shift-right: [w386] -> w337
                    shift-left: w367 -> [w387]
                    tunnel: [w385] -> w336 mode=indexing
                    n99 = Pick Line(multi-line string=w393, line index=w387) -> (output string=w391:string)  [unwired: 1 in]
                    n100 = Increment(x=w387) -> (x+1=w386:i32)
                    n101 = call "Numeric String to Bytes.vi"("Type"=T2."I8", "String"=w391) -> ("error out"=w385:errorcluster, "Byte Data"=w390:u8[])  [unwired: 8 in]
                    n102 = Build Array (concatenate)(w389, w390) -> (w388:u8[])
                  }
                  n103 = Replace Array Subset(array=w335, new element=w346, index=0) -> (w333:u8[])
                  n104 = call "Numeric String to Bytes.vi"("Type"=T2."U16", "String"=w381) -> ("error out"=w357:errorcluster, "Byte Data"=w365:u8[])  [unwired: 8 in]
                  n105 = call "Numeric String to Bytes.vi"("Type"=T2."U16", "String"=w382) -> ("error out"=w356:errorcluster, "Byte Data"=w364:u8[])  [unwired: 8 in]
                  n106 = call "Numeric String to Bytes.vi"("Type"=T2."I16", "String"=w375) -> ("error out"=w355:errorcluster, "Byte Data"=w363:u8[])  [unwired: 8 in]
                  n107 = call "Numeric String to Bytes.vi"("Type"=T2."U16", "String"=w376) -> ("error out"=w354:errorcluster, "Byte Data"=w362:u8[])  [unwired: 8 in]
                  n108 = call "Numeric String to Bytes.vi"("Type"=T2."U16", "String"=w377) -> ("error out"=w353:errorcluster, "Byte Data"=w361:u8[])  [unwired: 8 in]
                  n109 = call "Numeric String to Bytes.vi"("Type"=T2."U16", "String"=w373) -> ("error out"=w352:errorcluster, "Byte Data"=w360:u8[])  [unwired: 8 in]
                  n110 = Split 1D Array(array=w333, index=16) -> (first subarray=w332:u8[])  [unwired: 1 out]
                  n111 = Build Array (concatenate)(w366, w332, w365, w364, w363, w362, w361, w360, w359) -> (w349:u8[])
                  n112 = Build Array (concatenate)(w358, w357, w356, w355, w354, w353, w352, w336) -> (w350:errorcluster[])
                  n113 = Merge Errors(w350) -> (w351:errorcluster)
                }
              }
            }
            n114 = Unbundle By Name(w263) -> ("status"=w262:bool)
            n115 = Or(x=w261, y=w262) -> (x .or. y?=w260:bool)
          }
        }
        frame "Get Program Constants" {
          # "Get Program Constants"
        }
        frame "Set Program Constants" {
          w407 = u8[] []  # DATA
          # "Set Program Constants"
          n116 = Pick Line(multi-line string=w398, line index=0) -> (output string=w404:string)  [unwired: 1 in]
          n117 = for {
            N: 64 -> [_]
            tunnel: w398 -> [w420]
            shift-right: [w413] -> w406
            shift-left: w407 -> [w414]
            tunnel: 1 -> [w415]
            tunnel: [w411] -> w400 mode=indexing
            i -> [w417]
            n118 = Add(x=w415, y=w417) -> (x+y=w416:i32)
            n119 = Pick Line(multi-line string=w420, line index=w416) -> (output string=w419:string)  [unwired: 1 in]
            n120 = call "Numeric String to Bytes.vi"("Type"=T2."U16", "String"=w419) -> ("error out"=w411:errorcluster, "Byte Data"=w412:u8[])  [unwired: 8 in]
            n121 = Build Array (concatenate)(w414, w412) -> (w413:u8[])
          }
          n122 = call "Numeric String to Bytes.vi"("Type"=T2."U16", "String"=w404) -> ("error out"=w399:errorcluster, "Byte Data"=w402:u8[])  [unwired: 8 in]
          n123 = Build Array (concatenate)(w402, w406) -> (w408:u8[])
          n124 = Merge Errors(w399, w400) -> (w401:errorcluster)
        }
        frame "Get Configurable Device Parameters" {
          # "Get Configurable Device Parameters"
        }
        frame "Set Configurable Device Parameters" {
          w424 = u8[] [0] ("array")
          w446 = 0
          w490 = u8[] [0, 0, 0, 0, 0, 0, 0, 0, 0, 0, 0, 0, 0, 0, 0, 0, 0, 0, 0, 0, 0, 0, 0, 0, 0, 0, 0, 0, 0, 0]  # DATA
          w497 = u8[] []  # DATA
          # "Changed to U8 from U16"
          # "Set Configurable Device Parameters"
          n125 = Pick Line(multi-line string=w428, line index=17) -> (output string=w426:string)  [unwired: 1 in]
          n126 = Match Pattern(string=w426, regular expression="=") -> (after substring=w425:string)  [unwired: 1 in, 3 out]
          n127 = Scan From String(format string="%d/%d/%d %d=%d=%d %s", input string=w425) -> (error out=w444:errorcluster, output 1=w454:i32, output 2=w453:i32, output 3=w452:i32, output 4=w451:i32, output 5=w450:i32, output 6=w449:i32, output 7=w455:string)  [unwired: 9 in, 2 out]
          n128 = case shown="\"PM\"" w455 {
            tunnel: w451 -> [w499 w501 w504]
            tunnel: [w499 w500 w503] -> w448
            frame Default {
            }
            frame "AM" {
              n129 = Subtract(x=w501, y=12) -> (x-y=w500:i32)
            }
            frame "PM" {
              n130 = Add(x=w504, y=12) -> (x+y=w503:i32)
            }
          }
          n131 = for {
            N: 12 -> [_]
            tunnel: [w511] -> w489 mode=indexing
            tunnel: w428 -> [w510]
            shift-right: [w508] -> w484
            shift-left: w497 -> [w507]
            i -> [w509]
            n132 = Pick Line(multi-line string=w510, line index=w509) -> (output string=w512:string)  [unwired: 1 in]
            n133 = call "Numeric String to Bytes.vi"("Type"=T2."U8", "String"=w512) -> ("error out"=w511:errorcluster, "Byte Data"=w506:u8[])  [unwired: 8 in]
            n134 = Build Array (concatenate)(w507, w506) -> (w508:u8[])
          }
          n135 = Pick Line(multi-line string=w428, line index=12) -> (output string=w486:string)  [unwired: 1 in]
          n136 = Pick Line(multi-line string=w428, line index=13) -> (output string=w480:string)  [unwired: 1 in]
          n137 = Pick Line(multi-line string=w428, line index=14) -> (output string=w475:string)  [unwired: 1 in]
          n138 = Pick Line(multi-line string=w428, line index=15) -> (output string=w472:string)  [unwired: 1 in]
          n139 = Pick Line(multi-line string=w428, line index=16) -> (output string=w469:string)  [unwired: 1 in]
          n140 = Pick Line(multi-line string=w428, line index=18) -> (output string=w458:string)  [unwired: 1 in]
          n141 = Bundle By Name(cluster=T3 {"fractional second"=0.0, "second"=0, "minute"=0, "hour"=0, "day of month"=0, "month"=0, "year"=0, "day of week"=0, "day of year"=0, "DST"=0} ("date time rec"), "month"=w454, "day of month"=w453, "year"=w452, "hour"=w448, "minute"=w450, "second"=w449, "day of week"=w446, "day of year"=w446, "DST"=w446, "fractional second"=w446) -> (w445:T3)
          n142 = Match Pattern(string=w486, regular expression="=") -> (after substring=w485:string)  [unwired: 1 in, 3 out]
          n143 = call "Numeric String to Bytes.vi"("Type"=T2."U16", "String"=w480) -> ("error out"=w478:errorcluster, "Byte Data"=w479:u8[])  [unwired: 8 in]
          n144 = call "Numeric String to Bytes.vi"("Type"=T2."U8", "String"=w475) -> ("error out"=w467:errorcluster, "Byte Data"=w464:u8[])  [unwired: 8 in]
          n145 = call "Numeric String to Bytes.vi"("Type"=T2."U8", "String"=w472) -> ("error out"=w466:errorcluster, "Byte Data"=w463:u8[])  [unwired: 8 in]
          n146 = call "Numeric String to Bytes.vi"("Type"=T2."U8", "String"=w469) -> ("error out"=w465:errorcluster, "Byte Data"=w462:u8[])  [unwired: 8 in]
          n147 = call "Numeric String to Bytes.vi"("Type"=T2."U8", "String"=w458) -> ("error out"=w432:errorcluster, "Byte Data"=w459:u8[])  [unwired: 8 in]
          n148 = call <vilib>:"Trim Whitespace.vi"("string"=w485) -> ("trimmed string"=w493:string)  [unwired: 1 in]
          n149 = String To Byte Array(string=w493) -> (unsigned byte array=w492:u8[])
          n150 = Date/Time To Seconds(2:w445) -> (0:w441:timestamp)  [unwired: 1 in]
          n151 = Replace Array Subset(array=w490, new element=w492, index=0) -> (w482:u8[])
          n152 = To Unsigned Quad Integer(1:w441) -> (0:w440:u64)
          n153 = Multiply(x=u64 1904 ("y"), y=u64 31556926) -> (x*y=w439:u64)
          n154 = Add(x=w440, y=w439) -> (x+y=w438:u64)
          n155 = Multiply(x=u64 10000000 ("y"), y=w438) -> (x*y=w436:u64)
          n156 = Number To Decimal String(number=w436) -> (decimal integer string=w433:string)  [unwired: 1 in]
          n157 = Concatenate Strings("MS_Date=" ("string"), w433) -> (w434:string)
          n158 = call "Numeric String to Bytes.vi"("Type"=T2."U64", "String"=w434) -> ("error out"=w431:errorcluster, "Byte Data"=w429:u8[])  [unwired: 8 in]
          n159 = Build Array (concatenate)(w484, w482, w479, w464, w463, w462, w424, w429, w459, w424) -> (w495:u8[])
          n160 = Build Array (concatenate)(w489, w478, w467, w466, w465, w444, w431, w432) -> (w488:errorcluster[])
          n161 = Merge Errors(w488) -> (w496:errorcluster)
        }
        frame "Get Pulse Constants" {
          # "Get Pulse Constants"
        }
        frame "Set Pulse Constants" {
          w517 = u8[] []  # DATA
          # "Set Pulse Constants"
          n162 = for {
            N: 11 -> [_]
            tunnel: w522 -> [w542]
            shift-right: [w538] -> w533
            shift-left: w517 -> [w539]
            tunnel: [w536] -> w520 mode=indexing
            i -> [w543]
            n163 = Pick Line(multi-line string=w542, line index=w543) -> (output string=w541:string)  [unwired: 1 in]
            n164 = call "Numeric String to Bytes.vi"("Type"=T2."U16", "String"=w541) -> ("error out"=w536:errorcluster, "Byte Data"=w537:u8[])  [unwired: 8 in]
            n165 = Build Array (concatenate)(w539, w537) -> (w538:u8[])
          }
          n166 = Pick Line(multi-line string=w522, line index=11) -> (output string=w530:string)  [unwired: 1 in]
          n167 = Pick Line(multi-line string=w522, line index=12) -> (output string=w527:string)  [unwired: 1 in]
          n168 = call "Numeric String to Bytes.vi"("Type"=T2."U8", "String"=w530) -> ("error out"=w518:errorcluster, "Byte Data"=w523:u8[])  [unwired: 8 in]
          n169 = call "Numeric String to Bytes.vi"("Type"=T2."U8", "String"=w527) -> ("error out"=w521:errorcluster, "Byte Data"=w524:u8[])  [unwired: 8 in]
          n170 = Build Array (concatenate)(w533, w523, w524) -> (w532:u8[])
          n171 = Build Array (concatenate)(w520, w518, w521) -> (w519:errorcluster[])
          n172 = Merge Errors(w519) -> (w531:errorcluster)
        }
        frame "Get Lead Limits" {
          # "Get Lead Limits"
        }
        frame "Set Lead Limits" {
          w547 = u8[] []  # DATA
          # "Set Lead Limits"
          n173 = for {
            N: 52 -> [_]
            tunnel: w550 -> [w560]
            shift-right: [w556] -> w548
            shift-left: w547 -> [w557]
            tunnel: [w554] -> w549 mode=indexing
            i -> [w561]
            n174 = Pick Line(multi-line string=w560, line index=w561) -> (output string=w559:string)  [unwired: 1 in]
            n175 = call "Numeric String to Bytes.vi"("Type"=T2."U16", "String"=w559) -> ("error out"=w554:errorcluster, "Byte Data"=w555:u8[])  [unwired: 8 in]
            n176 = Build Array (concatenate)(w557, w555) -> (w556:u8[])
          }
          n177 = Merge Errors(w549) -> (w551:errorcluster)
        }
        frame "Get Channel Calibrations" {
          # "Get Channel Calibrations"
          n178 = call "Numeric String to Bytes.vi"("Type"=T2."U8", "String"=w564) -> ("error out"=w565:errorcluster, "Byte Data"=w567:u8[])  [unwired: 8 in]
          n179 = Replace Array Subset(array=w563, new element=w567, index=0) -> (w562:u8[])
        }
        frame "Set Channel Calibrations" {
          w578 = u8[] []  # DATA
          # "Set Channel Calibrations"
          n180 = for {
            N: 52 -> [_]
            tunnel: w571 -> [w591]
            shift-right: [w587] -> w573
            shift-left: w578 -> [w588]
            tunnel: [w585] -> w579 mode=indexing
            i -> [w583]
            n181 = Increment(x=w583) -> (x+1=w584:i32)
            n182 = Pick Line(multi-line string=w591, line index=w584) -> (output string=w590:string)  [unwired: 1 in]
            n183 = call "Numeric String to Bytes.vi"("Type"=T2."U16", "String"=w590) -> ("error out"=w585:errorcluster, "Byte Data"=w586:u8[])  [unwired: 8 in]
            n184 = Build Array (concatenate)(w588, w586) -> (w587:u8[])
          }
          n185 = Pick Line(multi-line string=w571, line index=0) -> (output string=w577:string)  [unwired: 1 in]
          n186 = call "Numeric String to Bytes.vi"("Type"=T2."U16", "String"=w577) -> ("error out"=w570:errorcluster, "Byte Data"=w572:u8[])  [unwired: 8 in]
          n187 = Build Array (concatenate)(w572, w573) -> (w574:u8[])
          n188 = Merge Errors(w579, w570) -> (w580:errorcluster)
        }
        frame "Get Stim Asic HV Calibrations" {
          # "Get Stim ASIC HV Calibrations"
        }
        frame "Set Stim Asic HV Calibrations" {
          w595 = u8[] []  # DATA
          # "Set Stim ASIC HV Calibrations"
          n189 = for {
            N: 64 -> [_]
            tunnel: w598 -> [w608]
            shift-right: [w604] -> w596
            shift-left: w595 -> [w605]
            tunnel: [w602] -> w597 mode=indexing
            i -> [w609]
            n190 = Pick Line(multi-line string=w608, line index=w609) -> (output string=w607:string)  [unwired: 1 in]
            n191 = call "Numeric String to Bytes.vi"("Type"=T2."U16", "String"=w607) -> ("error out"=w602:errorcluster, "Byte Data"=w603:u8[])  [unwired: 8 in]
            n192 = Build Array (concatenate)(w605, w603) -> (w604:u8[])
          }
          n193 = Merge Errors(w597) -> (w599:errorcluster)
        }
        frame "Get CP Data" {
          # "Get CP Data"
          n194 = call "Numeric String to Bytes.vi"("Type"=T2."U8", "String"=w615) -> ("error out"=w614:errorcluster, "Byte Data"=w611:u8[])  [unwired: 8 in]
          n195 = Replace Array Subset(array=w616, new element=w611, index=0) -> (w613:u8[])
        }
        frame "Set CP Data" {
          # "Set CP Data"
          n196 = Array To Cluster(array=w620) -> (cluster=w618:T4)
          n197 = Pick Line(multi-line string=w624, line index=0) -> (output string=w626:string)  [unwired: 1 in]
          n198 = Cluster To Array(cluster=w618) -> (array=w619:u8[])
          n199 = call "Numeric String to Bytes.vi"("Type"=T2."U16", "String"=w626) -> ("error out"=w621:errorcluster, "Byte Data"=w622:u8[])  [unwired: 8 in]
          n200 = Build Array (concatenate)(w622, w619) -> (w623:u8[])
          n201 = Merge Errors(w621) -> (w628:errorcluster)
        }
        frame "Clear Log" {
          # "Clear Log"
          n202 = call "Numeric String to Bytes.vi"("Type"=T2."U8", "String"=w635) -> ("error out"=w634:errorcluster, "Byte Data"=w631:u8[])  [unwired: 8 in]
          n203 = Replace Array Subset(array=w636, new element=w631, index=0) -> (w633:u8[])
        }
        frame "Read Log" {
          # "RESERVED (ALWAYS 0)"
          # "Read Log"
          n204 = Pick Line(multi-line string=w640, line index=0) -> (output string=w650:string)  [unwired: 1 in]
          n205 = Pick Line(multi-line string=w640, line index=1) -> (output string=w647:string)  [unwired: 1 in]
          n206 = call "Numeric String to Bytes.vi"("Type"=T2."U8", "String"=w650) -> ("error out"=w644:errorcluster, "Byte Data"=w639:u8[])  [unwired: 8 in]
          n207 = call "Numeric String to Bytes.vi"("Type"=T2."U32", "String"=w647) -> ("error out"=w643:errorcluster, "Byte Data"=w645:u8[])  [unwired: 8 in]
          n208 = Build Array (concatenate)(w639, u8[] [0] ("array"), w645) -> (w646:u8[])
          n209 = Build Array(w644, w643) -> (w642:errorcluster[])
          n210 = Replace Array Subset(array=w655, new element=w646, index=0) -> (w654:u8[])
          n211 = Merge Errors(w642) -> (w641:errorcluster)
        }
        frame "Append Log" {
          # "Added a U8 Data"
          # "Changed to U16 from U8"
          # "Append Log"
          n212 = Pick Line(multi-line string=w659, line index=0) -> (output string=w688:string)  [unwired: 1 in]
          n213 = Pick Line(multi-line string=w659, line index=1) -> (output string=w685:string)  [unwired: 1 in]
          n214 = Pick Line(multi-line string=w659, line index=2) -> (output string=w675:string)  [unwired: 1 in]
          n215 = Pick Line(multi-line string=w659, line index=3) -> (output string=w672:string)  [unwired: 1 in]
          n216 = Pick Line(multi-line string=w659, line index=4) -> (output string=w669:string)  [unwired: 1 in]
          n217 = Pick Line(multi-line string=w659, line index=5) -> (output string=w662:string)  [unwired: 1 in]
          n218 = call "Numeric String to Bytes.vi"("Type"=T2."U16", "String"=w688) -> ("error out"=w681:errorcluster, "Byte Data"=w684:u8[])  [unwired: 8 in]
          n219 = call "Numeric String to Bytes.vi"("Type"=T2."U16", "String"=w685) -> ("error out"=w680:errorcluster, "Byte Data"=w682:u8[])  [unwired: 8 in]
          n220 = call "Numeric String to Bytes.vi"("Type"=T2."U8", "String"=w675) -> ("error out"=w665:errorcluster, "Byte Data"=w666:u8[])  [unwired: 8 in]
          n221 = call "Numeric String to Bytes.vi"("Type"=T2."U8", "String"=w672) -> ("error out"=w664:errorcluster, "Byte Data"=w667:u8[])  [unwired: 8 in]
          n222 = call "Numeric String to Bytes.vi"("Type"=T2."U8", "String"=w669) -> ("error out"=w663:errorcluster, "Byte Data"=w668:u8[])  [unwired: 8 in]
          n223 = call "Numeric String to Bytes.vi"("Type"=T2."U8", "String"=w662) -> ("error out"=w658:errorcluster, "Byte Data"=w657:u8[])  [unwired: 8 in]
          n224 = Build Array (concatenate)(w684, w682, w666, w667, w668, w657) -> (w683:u8[])
          n225 = Build Array(w681, w680, w665, w664, w663, w658) -> (w679:errorcluster[])
          n226 = Replace Array Subset(array=w693, new element=w683, index=0) -> (w692:u8[])
          n227 = Merge Errors(w679) -> (w678:errorcluster)
        }
        frame "Get Patient Program Runtime" {
          # "Get Patient Program Run-Time"
          n228 = call "Numeric String to Bytes.vi"("Type"=T2."U8", "String"=w700) -> ("error out"=w699:errorcluster, "Byte Data"=w696:u8[])  [unwired: 8 in]
          n229 = Replace Array Subset(array=w701, new element=w696, index=0) -> (w698:u8[])
        }
        frame "Set Patient Program Runtime" {
          # "Set Patient Program Run-Time"
          n230 = Pick Line(multi-line string=w703, line index=0) -> (output string=w714:string)  [unwired: 1 in]
          n231 = Pick Line(multi-line string=w703, line index=1) -> (output string=w711:string)  [unwired: 1 in]
          n232 = call "Numeric String to Bytes.vi"("Type"=T2."U16", "String"=w714) -> ("error out"=w707:errorcluster, "Byte Data"=w710:u8[])  [unwired: 8 in]
          n233 = call "Numeric String to Bytes.vi"("Type"=T2."U32", "String"=w711) -> ("error out"=w706:errorcluster, "Byte Data"=w708:u8[])  [unwired: 8 in]
          n234 = Build Array (concatenate)(w710, w708) -> (w709:u8[])
          n235 = Build Array(w707, w706) -> (w705:errorcluster[])
          n236 = Replace Array Subset(array=w719, new element=w709, index=0) -> (w718:u8[])
          n237 = Merge Errors(w705) -> (w704:errorcluster)
        }
        frame "Impedance Measurement" {
          # "Changed to U16 from U8"
          # "Impedance Measurement"
          n238 = Pick Line(multi-line string=w721, line index=0) -> (output string=w737:string)  [unwired: 1 in]
          n239 = Pick Line(multi-line string=w721, line index=1) -> (output string=w734:string)  [unwired: 1 in]
          n240 = Pick Line(multi-line string=w721, line index=2) -> (output string=w724:string)  [unwired: 1 in]
          n241 = call "Numeric String to Bytes.vi"("Type"=T2."U8", "String"=w737) -> ("error out"=w730:errorcluster, "Byte Data"=w733:u8[])  [unwired: 8 in]
          n242 = call "Numeric String to Bytes.vi"("Type"=T2."U8", "String"=w734) -> ("error out"=w729:errorcluster, "Byte Data"=w731:u8[])  [unwired: 8 in]
          n243 = call "Numeric String to Bytes.vi"("Type"=T2."U8", "String"=w724) -> ("error out"=w722:errorcluster, "Byte Data"=w723:u8[])  [unwired: 8 in]
          n244 = Build Array (concatenate)(w733, w731, w723) -> (w732:u8[])
          n245 = Replace Array Subset(array=w742, new element=w732, index=0) -> (w741:u8[])
          n246 = Build Array(w730, w729, w722) -> (w728:errorcluster[])
          n247 = Merge Errors(w728) -> (w727:errorcluster)
        }
        frame "Enter Storage Mode" {
          # "Enter Storage Mode"
        }
        frame "Echo Short" {
          # "Echo Short"
          n248 = Array Subset(array=w751, index=0, length=8) -> (w748:u8[])
        }
        frame "Echo Long" {
          # "Echo Long"
          n249 = Array Subset(array=w757, index=0, length=256) -> (w754:u8[])
        }
        frame "Get General Calibration" {
          # "Get General Calibration"
        }
        frame "Set General Calibration" {
          w762 = u8[] []  # DATA
          # "Set General Calibration"
          n250 = disable-structure shown="Disabled" {
            disable-tunnel: [w799 w851] -> w766
            disable-tunnel: [w795 w850] -> w764
            disable-tunnel: w763 -> [w782 w853]
            disable-tunnel: w762 -> [w768 w852]
            frame Disabled {
              n251 = for {
                N: 15 -> [_]
                tunnel: [w846] -> w800 mode=indexing
                tunnel: w782 -> [w845]
                shift-right: [w842] -> w794
                shift-left: w768 -> [w843]
                tunnel: [w841] -> w778
                i -> [w841]
                n252 = Pick Line(multi-line string=w845, line index=w841) -> (output string=w847:string)  [unwired: 1 in]
                n253 = call "Numeric String to Bytes.vi"("Type"=T2."U16", "String"=w847) -> ("error out"=w846:errorcluster, "Byte Data"=w844:u8[])  [unwired: 8 in]
                n254 = Build Array (concatenate)(w843, w844) -> (w842:u8[])
              }
              n255 = Increment(x=w778) -> (x+1=w777:i32)
              n256 = for {
                N: 12 -> [_]
                tunnel: [w808] -> w780 mode=indexing
                tunnel: w782 -> [w807]
                shift-right: [w804] -> w779
                shift-left: w768 -> [w805]
                tunnel: w777 -> [w802]
                tunnel: [w801] -> w775
                i -> [w801]
                n257 = Add(x=w802, y=w801) -> (x+y=w803:i32)
                n258 = Pick Line(multi-line string=w807, line index=w803) -> (output string=w809:string)  [unwired: 1 in]
                n259 = call "Numeric String to Bytes.vi"("Type"=T2."U16", "String"=w809) -> ("error out"=w808:errorcluster, "Byte Data"=w806:u8[])  [unwired: 8 in]
                n260 = Build Array (concatenate)(w805, w806) -> (w804:u8[])
              }
              n261 = Increment(x=w775) -> (x+1=w776:i32)
              n262 = for {
                N: 15 -> [_]
                tunnel: [w838] -> w792 mode=indexing
                tunnel: w782 -> [w837]
                shift-right: [w834] -> w793
                shift-left: w768 -> [w835]
                tunnel: w776 -> [w832]
                tunnel: [w831] -> w774
                i -> [w831]
                n263 = Add(x=w832, y=w831) -> (x+y=w833:i32)
                n264 = Pick Line(multi-line string=w837, line index=w833) -> (output string=w839:string)  [unwired: 1 in]
                n265 = call "Numeric String to Bytes.vi"("Type"=T2."U16", "String"=w839) -> ("error out"=w838:errorcluster, "Byte Data"=w836:u8[])  [unwired: 8 in]
                n266 = Build Array (concatenate)(w835, w836) -> (w834:u8[])
              }
              n267 = Increment(x=w774) -> (x+1=w773:i32)
              n268 = for {
                N: 5 -> [_]
                tunnel: [w828] -> w789 mode=indexing
                tunnel: w782 -> [w827]
                shift-right: [w824] -> w790
                shift-left: w768 -> [w825]
                tunnel: w773 -> [w822]
                tunnel: [w821] -> w771
                i -> [w821]
                n269 = Add(x=w822, y=w821) -> (x+y=w823:i32)
                n270 = Pick Line(multi-line string=w827, line index=w823) -> (output string=w829:string)  [unwired: 1 in]
                n271 = call "Numeric String to Bytes.vi"("Type"=T2."U16", "String"=w829) -> ("error out"=w828:errorcluster, "Byte Data"=w826:u8[])  [unwired: 8 in]
                n272 = Build Array (concatenate)(w825, w826) -> (w824:u8[])
              }
              n273 = Increment(x=w771) -> (x+1=w772:i32)
              n274 = for {
                N: 5 -> [_]
                tunnel: [w818] -> w786 mode=indexing
                tunnel: w782 -> [w817]
                shift-right: [w814] -> w787
                shift-left: _ -> [w815]
                tunnel: w772 -> [w812]
                tunnel: [w811] -> w770
                i -> [w811]
                n275 = Add(x=w812, y=w811) -> (x+y=w813:i32)
                n276 = Pick Line(multi-line string=w817, line index=w813) -> (output string=w819:string)  [unwired: 1 in]
                n277 = call "Numeric String to Bytes.vi"("Type"=T2."U16", "String"=w819) -> ("error out"=w818:errorcluster, "Byte Data"=w816:u8[])  [unwired: 8 in]
                n278 = Build Array (concatenate)(w815, w816) -> (w814:u8[])
              }
              n279 = Increment(x=w770) -> (x+1=w769:i32)
              n280 = Pick Line(multi-line string=w782, line index=w769) -> (output string=w797:string)  [unwired: 1 in]
              n281 = call "Numeric String to Bytes.vi"("Type"=T2."U16", "String"=w797) -> ("error out"=w785:errorcluster, "Byte Data"=w784:u8[])  [unwired: 8 in]
              n282 = Build Array (concatenate)(w794, w779, w793, w790, w787, w784) -> (w795:u8[])
              n283 = Build Array (concatenate)(w800, w780, w792, w789, w786, w785) -> (w799:errorcluster[])
            }
            frame Enabled {
              n284 = for {
                N: 55 -> [_]
                tunnel: [w859] -> w851 mode=indexing
                tunnel: w853 -> [w858]
                shift-right: [w855] -> w850
                shift-left: w852 -> [w856]
                i -> [w854]
                n285 = Pick Line(multi-line string=w858, line index=w854) -> (output string=w860:string)  [unwired: 1 in]
                n286 = call "Numeric String to Bytes.vi"("Type"=T2."U16", "String"=w860) -> ("error out"=w859:errorcluster, "Byte Data"=w857:u8[])  [unwired: 8 in]
                n287 = Build Array (concatenate)(w856, w857) -> (w855:u8[])
              }
            }
          }
          n288 = Merge Errors(w766) -> (w765:errorcluster)
        }
        frame "Get Trim List" {
          # "Changed to U8 from U16"
          # "Get Trim List"
          n289 = call "Numeric String to Bytes.vi"("Type"=T2."U8", "String"=w864) -> ("error out"=w863:errorcluster, "Byte Data"=w867:u8[])  [unwired: 8 in]
          n290 = Replace Array Subset(array=w865, new element=w867, index=0) -> (w862:u8[])
        }
        frame "Set Trim List" {
          w892 = u8[] []  # DATA
          # "Set Trim List"
          n291 = Pick Line(multi-line string=w873, line index=0) -> (output string=w891:string)  [unwired: 1 in]
          n292 = Pick Line(multi-line string=w873, line index=1) -> (output string=w889:string)  [unwired: 1 in]
          n293 = call "Numeric String to Bytes.vi"("Type"=T2."U8", "String"=w891) -> ("error out"=w879:errorcluster, "Byte Data"=w875:u8[])  [unwired: 8 in]
          n294 = call "Numeric String to Bytes.vi"("Type"=T2."U8", "String"=w889) -> ("error out"=w878:errorcluster, "Byte Data"=w887:u8[])  [unwired: 8 in]
          n295 = Index Array(array=w875, index=0) -> (element=w874:u8)
          n296 = Index Array(array=w887, index=0) -> (element=w886:u8)
          n297 = case shown="0, Default" w874 {
            tunnel: w892 -> [w905 w933]
            tunnel: w886 -> [w893 w923]
            tunnel: w873 -> [w904 w932]
            tunnel: [w903 w931] -> w882
            tunnel: [w902 w931] -> w880
            tunnel: [w898 w929] -> w877
            frame 0, Default {
              # "\"Normal\" Trim List, with Address:Data tuples"
              n298 = for {
                N: w893 -> [_]
                tunnel: w904 -> [w906]
                shift-right: [w919] -> w899
                shift-left: w905 -> [w920]
                tunnel: [w917] -> w903 mode=indexing
                tunnel: [w914] -> w902 mode=indexing
                i -> [w908]
                w909 = 2 ("y")
                n299 = Multiply(x=w909, y=w908) -> (x*y=w910:i32)
                n300 = Add(x=w909, y=w910) -> (x+y=w913:i32)
                n301 = Add(x=w910, y=3) -> (x+y=w912:i32)
                n302 = Pick Line(multi-line string=w906, line index=w913) -> (output string=w922:string)  [unwired: 1 in]
                n303 = Pick Line(multi-line string=w906, line index=w912) -> (output string=w916:string)  [unwired: 1 in]
                n304 = call "Numeric String to Bytes.vi"("Type"=T2."U16", "String"=w922) -> ("error out"=w917:errorcluster, "Byte Data"=w918:u8[])  [unwired: 8 in]
                n305 = call "Numeric String to Bytes.vi"("Type"=T2."U8", "String"=w916) -> ("error out"=w914:errorcluster, "Byte Data"=w907:u8[])  [unwired: 8 in]
                n306 = Build Array (concatenate)(w920, w918, w907) -> (w919:u8[])
              }
              n307 = Multiply(x=u8 3, y=w893) -> (x*y=w895:u8)
              n308 = Subtract(x=u8 96, y=w895) -> (x-y=w900:u8)
              n309 = Initialize Array(u8 0, w900) -> (w897:u8[])
              n310 = Build Array (concatenate)(w899, w897) -> (w898:u8[])
            }
            frame 2 {
              n311 = Decrement(x=w923) -> (x-1=w930:u8)
              n312 = for {
                N: w930 -> [_]
                tunnel: w932 -> [w937]
                shift-right: [w942] -> w928
                shift-left: w933 -> [w943]
                tunnel: [w940] -> w931 mode=indexing
                i -> [w936]
                # "\"Stim Trims\" List - Five U8's and a U16"
                n313 = Add(x=2 ("y"), y=w936) -> (x+y=w939:i32)
                n314 = Equal?(x=w936, y=5) -> (x = y?=w934:bool)
                n315 = Pick Line(multi-line string=w937, line index=w939) -> (output string=w944:string)  [unwired: 1 in]
                n316 = case shown="True" w934 {
                  tunnel: w944 -> [w947 w953]
                  tunnel: [w946 w949] -> w941
                  tunnel: [w945 w951] -> w940
                  frame False {
                    # "U8 Stim Trim"
                    n317 = call "Numeric String to Bytes.vi"("Type"=T2."U8", "String"=w947) -> ("error out"=w945:errorcluster, "Byte Data"=w946:u8[])  [unwired: 8 in]
                  }
                  frame True {
                    # "U16 Gain Trim"
                    n318 = call "Numeric String to Bytes.vi"("Type"=T2."U16", "String"=w953) -> ("error out"=w951:errorcluster, "Byte Data"=w950:u8[])  [unwired: 8 in]
                    n319 = Reverse 1D Array(array=w950) -> (reversed array=w949:u8[])
                  }
                }
                n320 = Build Array (concatenate)(w943, w941) -> (w942:u8[])
              }
              n321 = Subtract(x=96, y=w923) -> (x-y=w924:i32)
              n322 = Initialize Array(u8 0, w924) -> (w926:u8[])
              n323 = Build Array (concatenate)(w928, w926) -> (w929:u8[])
            }
          }
          n324 = Build Array (concatenate)(w875, w887, w877) -> (w872:u8[])
          n325 = Build Array (concatenate)(w882, w880, w879, w878) -> (w881:errorcluster[])
          n326 = Merge Errors(w881) -> (w870:errorcluster)
        }
        frame "Get Counter" {
          # "Get Counter"
          n327 = call "Numeric String to Bytes.vi"("Type"=T2."U8", "String"=w959) -> ("error out"=w958:errorcluster, "Byte Data"=w955:u8[])  [unwired: 8 in]
          n328 = Replace Array Subset(array=w960, new element=w955, index=0) -> (w957:u8[])
        }
        frame "Set Counter" {
          # "Set Counter"
          n329 = Pick Line(multi-line string=w964, line index=0) -> (output string=w974:string)  [unwired: 1 in]
          n330 = Pick Line(multi-line string=w964, line index=1) -> (output string=w971:string)  [unwired: 1 in]
          n331 = call "Numeric String to Bytes.vi"("Type"=T2."U8", "String"=w974) -> ("error out"=w968:errorcluster, "Byte Data"=w963:u8[])  [unwired: 8 in]
          n332 = call "Numeric String to Bytes.vi"("Type"=T2."U32", "String"=w971) -> ("error out"=w967:errorcluster, "Byte Data"=w969:u8[])  [unwired: 8 in]
          n333 = Build Array (concatenate)(w963, u8[] [0] ("array"), w969) -> (w970:u8[])
          n334 = Build Array(w968, w967) -> (w966:errorcluster[])
          n335 = Replace Array Subset(array=w979, new element=w970, index=0) -> (w978:u8[])
          n336 = Merge Errors(w966) -> (w965:errorcluster)
        }
        frame "Get Test Stimulation" {
          # "Get Test Stimulation"
        }
        frame "Set Test Stimulation" {
          w1001 = u8[] []  # DATA
          # "Set Test Stimulation"
          n337 = for {
            N: 4 -> [_]
            shift-right: [w1047] -> w985
            shift-left: w1001 -> [w1049]
            tunnel: w989 -> [w1026]
            shift-right: [w1022] -> _
            shift-left: 3 ("line index") -> [w1052]
            tunnel: [w1044] -> w1006 mode=indexing
            w1045 = u8[] []  # DATA
            n338 = Increment(x=w1052) -> (x+1=w1043:i32)
            n339 = Pick Line(multi-line string=w1026, line index=w1052) -> (output string=w1050:string)  [unwired: 1 in]
            n340 = for {
              N: 26 -> [_]
              tunnel: w1026 -> [w1061]
              shift-right: [w1056] -> w1024
              shift-left: w1045 -> [w1057]
              shift-right: [w1054] -> w1034
              shift-left: w1043 -> [w1055]
              tunnel: [w1053] -> _ mode=indexing
              n341 = Pick Line(multi-line string=w1061, line index=w1055) -> (output string=w1059:string)  [unwired: 1 in]
              n342 = Increment(x=w1055) -> (x+1=w1054:i32)
              n343 = call "Numeric String to Bytes.vi"("Type"=T2."I8", "String"=w1059) -> ("error out"=w1053:errorcluster, "Byte Data"=w1058:u8[])  [unwired: 8 in]
              n344 = Build Array (concatenate)(w1057, w1058) -> (w1056:u8[])
            }
            n345 = Increment(x=w1034) -> (x+1=w1033:i32)
            n346 = Pick Line(multi-line string=w1026, line index=w1034) -> (output string=w1042:string)  [unwired: 1 in]
            n347 = Increment(x=w1033) -> (x+1=w1032:i32)
            n348 = Pick Line(multi-line string=w1026, line index=w1033) -> (output string=w1039:string)  [unwired: 1 in]
            n349 = Increment(x=w1032) -> (x+1=w1030:i32)
            n350 = Pick Line(multi-line string=w1026, line index=w1032) -> (output string=w1037:string)  [unwired: 1 in]
            n351 = Increment(x=w1030) -> (x+1=w1025:i32)
            n352 = Pick Line(multi-line string=w1026, line index=w1030) -> (output string=w1036:string)  [unwired: 1 in]
            n353 = call "Numeric String to Bytes.vi"("Type"=T2."U16", "String"=w1050) -> ("error out"=w1015:errorcluster, "Byte Data"=w1048:u8[])  [unwired: 8 in]
            n354 = Increment(x=w1025) -> (x+1=w1023:i32)
            n355 = Pick Line(multi-line string=w1026, line index=w1025) -> (output string=w1035:string)  [unwired: 1 in]
            n356 = Pick Line(multi-line string=w1026, line index=w1023) -> (output string=w1027:string)  [unwired: 1 in]
            n357 = call "Numeric String to Bytes.vi"("Type"=T2."U16", "String"=w1042) -> ("error out"=w1014:errorcluster, "Byte Data"=w1021:u8[])  [unwired: 8 in]
            n358 = call "Numeric String to Bytes.vi"("Type"=T2."U8", "String"=w1039) -> ("error out"=w1013:errorcluster, "Byte Data"=w1020:u8[])  [unwired: 8 in]
            n359 = call "Numeric String to Bytes.vi"("Type"=T2."U8", "String"=w1037) -> ("error out"=w1012:errorcluster, "Byte Data"=w1019:u8[])  [unwired: 8 in]
            n360 = call "Numeric String to Bytes.vi"("Type"=T2."U16", "String"=w1036) -> ("error out"=w1011:errorcluster, "Byte Data"=w1018:u8[])  [unwired: 8 in]
            n361 = call "Numeric String to Bytes.vi"("Type"=T2."U16", "String"=w1035) -> ("error out"=w1010:errorcluster, "Byte Data"=w1017:u8[])  [unwired: 8 in]
            n362 = call "Numeric String to Bytes.vi"("Type"=T2."U8", "String"=w1027) -> ("error out"=w1009:errorcluster, "Byte Data"=w1016:u8[])  [unwired: 8 in]
            n363 = Build Array (concatenate)(w1049, w1048, w1024, w1021, w1020, w1019, w1018, w1017, w1016, u8[] [0] ("array")) -> (w1047:u8[])
            n364 = Merge Errors(w1015, w1014, w1013, w1012, w1011, w1010, w1009) -> (w1044:errorcluster)
            n365 = Increment(x=w1023) -> (x+1=w1022:i32)
          }
          n366 = Pick Line(multi-line string=w989, line index=2) -> (output string=w990:string)  [unwired: 1 in]
          n367 = Pick Line(multi-line string=w989, line index=0) -> (output string=w996:string)  [unwired: 1 in]
          n368 = Pick Line(multi-line string=w989, line index=1) -> (output string=w999:string)  [unwired: 1 in]
          n369 = call "Numeric String to Bytes.vi"("Type"=T2."U8", "String"=w990) -> ("Byte Data"=w988:u8[])  [unwired: 8 in, 1 out]
          n370 = call "Numeric String to Bytes.vi"("Type"=T2."U8", "String"=w996) -> ("error out"=w1004:errorcluster, "Byte Data"=w993:u8[])  [unwired: 8 in]
          n371 = call "Numeric String to Bytes.vi"("Type"=T2."U8", "String"=w999) -> ("error out"=w1005:errorcluster, "Byte Data"=w1003:u8[])  [unwired: 8 in]
          n372 = Build Array (concatenate)(w993, w1003, w988, u8[] [0] ("array"), w985) -> (w986:u8[])
          n373 = Merge Errors(w1004, w1005, w1006) -> (w987:errorcluster)
        }
        frame "Get Titration Stimulation" {
          # "Get Titration Stimulation"
        }
        frame "Set Titration Stimulation" {
          w1075 = u8[] []  # DATA
          # "Set Titration Stimulation"
          n374 = for {
            N: 4 -> [_]
            shift-right: [w1095] -> w1070
            shift-left: w1075 -> [w1098]
            tunnel: w1074 -> [w1084]
            shift-right: [w1089] -> _
            shift-left: 2 ("line index") -> [w1103]
            tunnel: [w1085] -> w1066 mode=indexing
            w1091 = u8[] []  # DATA
            n375 = Increment(x=w1103) -> (x+1=w1093:i32)
            n376 = Pick Line(multi-line string=w1084, line index=w1103) -> (output string=w1100:string)  [unwired: 1 in]
            n377 = Pick Line(multi-line string=w1084, line index=w1093) -> (output string=w1099:string)  [unwired: 1 in]
            n378 = Increment(x=w1093) -> (x+1=w1092:i32)
            n379 = call "Numeric String to Bytes.vi"("Type"=T2."U16", "String"=w1100) -> ("error out"=w1088:errorcluster, "Byte Data"=w1097:u8[])  [unwired: 8 in]
            n380 = call "Numeric String to Bytes.vi"("Type"=T2."U16", "String"=w1099) -> ("error out"=w1087:errorcluster, "Byte Data"=w1096:u8[])  [unwired: 8 in]
            n381 = for {
              N: 26 -> [_]
              tunnel: w1084 -> [w1112]
              shift-right: [w1107] -> w1090
              shift-left: w1091 -> [w1108]
              shift-right: [w1105] -> w1089
              shift-left: w1092 -> [w1106]
              tunnel: [w1104] -> w1086 mode=indexing
              n382 = Pick Line(multi-line string=w1112, line index=w1106) -> (output string=w1110:string)  [unwired: 1 in]
              n383 = Increment(x=w1106) -> (x+1=w1105:i32)
              n384 = call "Numeric String to Bytes.vi"("Type"=T2."I8", "String"=w1110) -> ("error out"=w1104:errorcluster, "Byte Data"=w1109:u8[])  [unwired: 8 in]
              n385 = Build Array (concatenate)(w1108, w1109) -> (w1107:u8[])
            }
            n386 = Build Array (concatenate)(w1098, w1097, w1096, w1090) -> (w1095:u8[])
            n387 = Merge Errors(w1088, w1087, w1086) -> (w1085:errorcluster)
          }
          n388 = Pick Line(multi-line string=w1074, line index=0) -> (output string=w1080:string)  [unwired: 1 in]
          n389 = Pick Line(multi-line string=w1074, line index=1) -> (output string=w1077:string)  [unwired: 1 in]
          n390 = call "Numeric String to Bytes.vi"("Type"=T2."U8", "String"=w1080) -> ("error out"=w1068:errorcluster, "Byte Data"=w1072:u8[])  [unwired: 8 in]
          n391 = call "Numeric String to Bytes.vi"("Type"=T2."U8", "String"=w1077) -> ("error out"=w1067:errorcluster, "Byte Data"=w1071:u8[])  [unwired: 8 in]
          n392 = Build Array (concatenate)(w1072, w1071, w1070) -> (w1069:u8[])
          n393 = Merge Errors(w1068, w1067, w1066) -> (w1065:errorcluster)
        }
        frame "Get Ramp Time" {
          # "Get Ramp Time"
        }
        frame "Set Ramp Time" {
          # "Set Ramp Time"
          n394 = call "Numeric String to Bytes.vi"("Type"=T2."U16", "String"=w1120) -> ("error out"=w1116:errorcluster, "Byte Data"=w1118:u8[])  [unwired: 8 in]
          n395 = Replace Array Subset(array=w1119, new element=w1118, index=0) -> (w1117:u8[])
        }
        frame "Get VBAT" {
          # "Get VBAT"
        }
        frame "Set Software Description Block" {
          # "Set Software Description Block"
        }
        frame "Get Software Description Block" {
          # "Get Software Description Block"
        }
        frame "Write Memory" {
          # "Write Memory"
          n396 = Initialize Array(u8 0 ("index"), 64 ("dimension size")) -> (w1135:u8[])
          n397 = Pick Line(multi-line string=w1143, line index=0) -> (output string=w1151:string)  [unwired: 1 in]
          n398 = Pick Line(multi-line string=w1143, line index=1) -> (output string=w1148:string)  [unwired: 1 in]
          n399 = Build Array (concatenate)(w1134, w1135) -> (w1133:u8[])
          n400 = call "Numeric String to Bytes.vi"("Type"=T2."U32", "String"=w1151) -> ("error out"=w1145:errorcluster, "Byte Data"=w1147:u8[])  [unwired: 8 in]
          n401 = call "Numeric String to Bytes.vi"("Type"=T2."U16", "String"=w1148) -> ("error out"=w1144:errorcluster, "Byte Data"=w1146:u8[])  [unwired: 8 in]
          n402 = Merge Errors(w1145, w1144) -> (w1141:errorcluster)
          n403 = Array Subset(array=w1133, index=0, length=64) -> (w1138:u8[])
          n404 = Build Array (concatenate)(w1147, w1146, w1138) -> (w1142:u8[])
        }
        frame "Read Memory" {
          # "Read Memory"
          n405 = Pick Line(multi-line string=w1166, line index=0) -> (output string=w1168:string)  [unwired: 1 in]
          n406 = Pick Line(multi-line string=w1166, line index=1) -> (output string=w1164:string)  [unwired: 1 in]
          n407 = call "Numeric String to Bytes.vi"("Type"=T2."U32", "String"=w1168) -> ("error out"=w1159:errorcluster, "Byte Data"=w1161:u8[])  [unwired: 8 in]
          n408 = call "Numeric String to Bytes.vi"("Type"=T2."U16", "String"=w1164) -> ("error out"=w1158:errorcluster, "Byte Data"=w1160:u8[])  [unwired: 8 in]
          n409 = Build Array (concatenate)(w1161, w1160) -> (w1162:u8[])
          n410 = Merge Errors(w1159, w1158) -> (w1157:errorcluster)
          n411 = Replace Array Subset(array=w1156, new element=w1162, index=0) -> (w1155:u8[])
        }
        frame "Reset xPG" {
          # "Reset xPG"
        }
        frame "Erase Flash Block" {
          # "Erase Flash Block"
        }
        frame "Write Vectors" {
          # "Write Vectors"
        }
        frame "Read Vectors" {
          # "Read Vectors"
        }
        frame "Diagnostic Data" {
          # "Diagnostic  Data"
          n412 = Pick Line(multi-line string=w1196, line index=0) -> (output string=w1197:string)  [unwired: 1 in]
          n413 = Pick Line(multi-line string=w1196, line index=1) -> (output string=w1193:string)  [unwired: 1 in]
          n414 = call "Numeric String to Bytes.vi"("Type"=T2."U8", "String"=w1197) -> ("error out"=w1190:errorcluster, "Byte Data"=w1192:u8[])  [unwired: 8 in]
          n415 = call "Numeric String to Bytes.vi"("Type"=T2."U8", "String"=w1193) -> ("error out"=w1189:errorcluster, "Byte Data"=w1191:u8[])  [unwired: 8 in]
          n416 = Build Array (concatenate)(w1192, w1191) -> (w1185:u8[])
          n417 = Merge Errors(w1190, w1189) -> (w1188:errorcluster)
          n418 = Replace Array Subset(array=w1187, new element=w1185, index=0) -> (w1184:u8[])
        }
        frame "Set Background Impedance" {
          # "Set Background Impedance"
          n419 = Pick Line(multi-line string=w1204, line index=0) -> (output string=w1207:string)  [unwired: 1 in]
          n420 = Pick Line(multi-line string=w1204, line index=1) -> (output string=w1205:string)  [unwired: 1 in]
          n421 = call "Numeric String to Bytes.vi"("Type"=T2."U8", "String"=w1207) -> ("error out"=w1203:errorcluster, "Byte Data"=w1212:u8[])  [unwired: 8 in]
          n422 = call "Numeric String to Bytes.vi"("Type"=T2."U8", "String"=w1205) -> ("error out"=w1202:errorcluster, "Byte Data"=w1210:u8[])  [unwired: 8 in]
          n423 = Build Array (concatenate)(w1212, w1210) -> (w1209:u8[])
          n424 = Merge Errors(w1203, w1202) -> (w1201:errorcluster)
        }
        frame "Inject Event" {
          # "Inject Event"
          n425 = Pick Line(multi-line string=w1218, line index=0) -> (output string=w1221:string)  [unwired: 1 in]
          n426 = Pick Line(multi-line string=w1218, line index=1) -> (output string=w1219:string)  [unwired: 1 in]
          n427 = call "Numeric String to Bytes.vi"("Type"=T2."U16", "String"=w1221) -> ("error out"=w1217:errorcluster, "Byte Data"=w1226:u8[])  [unwired: 8 in]
          n428 = call "Numeric String to Bytes.vi"("Type"=T2."U16", "String"=w1219) -> ("error out"=w1216:errorcluster, "Byte Data"=w1224:u8[])  [unwired: 8 in]
          n429 = Build Array (concatenate)(w1226, w1224) -> (w1223:u8[])
          n430 = Merge Errors(w1217, w1216) -> (w1215:errorcluster)
        }
        frame "Get Background Impedence " {
          # "Get Background Impedance"
        }
        frame "Set Test Waveform" {
        }
        frame "Calibrate Channel" {
        }
        frame "Get Log Range" {
          n431 = Pick Line(multi-line string=w1245, line index=0) -> (output string=w1243:string)  [unwired: 1 in]
          n432 = call "Numeric String to Bytes.vi"("Type"=T2."U8", "String"=w1243) -> ("error out"=w1238:errorcluster, "Byte Data"=w1240:u8[])  [unwired: 8 in]
          n433 = Replace Array Subset(array=w1241, new element=w1240, index=0) -> (w1239:u8[])
        }
        frame "Reserved 0x55" {
        }
        frame "Reserved 0x56" {
        }
        frame "MICS Options" {
        }
        frame "Pair PPC" {
        }
        frame "Pair POP" {
        }
        frame "Stop Bootloader" {
        }
        frame "Tune MICS" {
        }
        frame "MICS Diagnostics" {
          # "Added extra U8 to match xCT"
          # "Diagnostic Mode"
          # "Duration"
          # "Delay"
          # "Channel"
          n434 = Pick Line(multi-line string=w1287, line index=0) -> (output string=w1286:string)  [unwired: 1 in]
          n435 = Pick Line(multi-line string=w1287, line index=1) -> (output string=w1285:string)  [unwired: 1 in]
          n436 = Pick Line(multi-line string=w1287, line index=2) -> (output string=w1284:string)  [unwired: 1 in]
          n437 = Pick Line(multi-line string=w1287, line index=3) -> (output string=w1283:string)  [unwired: 1 in]
          n438 = call "Numeric String to Bytes.vi"("Type"=T2."U8", "String"=w1286) -> ("error out"=w1278:errorcluster, "Byte Data"=w1282:u8[])  [unwired: 8 in]
          n439 = call "Numeric String to Bytes.vi"("Type"=T2."U16", "String"=w1285) -> ("error out"=w1277:errorcluster, "Byte Data"=w1281:u8[])  [unwired: 8 in]
          n440 = call "Numeric String to Bytes.vi"("Type"=T2."U16", "String"=w1284) -> ("error out"=w1276:errorcluster, "Byte Data"=w1280:u8[])  [unwired: 8 in]
          n441 = call "Numeric String to Bytes.vi"("Type"=T2."U8", "String"=w1283) -> ("error out"=w1275:errorcluster, "Byte Data"=w1279:u8[])  [unwired: 8 in]
          n442 = Build Array (concatenate)(u8[] [0] ("array"), w1282, w1281, w1280, w1279) -> (w1273:u8[])
          n443 = Merge Errors(w1278, w1277, w1276, w1275) -> (w1274:errorcluster)
          n444 = Replace Array Subset(array=w1272, new element=w1273, index=0) -> (w1271:u8[])
        }
        frame "Undefined" {
        }
        frame "<reserved 2>" {
        }
        frame "<reserved 3>" {
        }
        frame "<reserved 4>" {
        }
        frame "<reserved 5>" {
        }
        frame "<reserved 6>" {
        }
        frame "<reserved 7>" {
        }
        frame "<reserved 8>" {
        }
        frame "<reserved 9>" {
        }
      }
      n445 = Increment(x=w15) -> (x+1=w3:T1)
      n446 = while {
        tunnel: w3 -> [w20]
        tunnel: "EXID" -> [w19]
        shift-right: [w21] -> _
        shift-left: w13 -> [w22]
        tunnel: w10 -> [w17]
        tunnel: [w16] -> w12 mode=indexing
        i -> [w23]
        stop <- w18 continue-if-true
        n447 = case shown="1, Default" w23 {
          tunnel: w22 -> [w46 w56]
          tunnel: [w45 w60] -> w21
          tunnel: w20 -> [w26 _]
          tunnel: w19 -> [w42 _]
          tunnel: [w43 w58] -> w18
          tunnel: w17 -> [w38 w50]
          tunnel: [w29 w52] -> w16
          frame 0 {
            n448 = Split Number(x=w42) -> (hi(x)=w41:u16, lo(x)=w40:u16)
            n449 = Array To Cluster(array=w38) -> (cluster=w39:T5)
            n450 = Split Number(x=w41) -> (lo(x)=w36:u8)  [unwired: 1 out]
            n451 = Split Number(x=w40) -> (hi(x)=w37:u8, lo(x)=w35:u8)
            n452 = Delete From Array(array=w46, length=8, index=0) -> (deleted portion=w31:u8[], array with subset deleted=w45:u8[])
            n453 = Split Number(x=w26) -> (hi(x)=w27:u8, lo(x)=w28:u8)
            n454 = Bundle By Name(cluster=w39, "DATA[5]"=w27, "DATA[4]"=w28, "DATA[3]"=w36, "DATA[2]"=w37, "DATA[1]"=w35, "DATA[0]"=1) -> (w33:T5)
            n455 = Cluster To Array(cluster=w33) -> (array=w30:u8[])
            n456 = Array Size(array=w45) -> (size(s)=w44:i32)
            n457 = Replace Array Subset(array=w30, new element=w31, index=6) -> (w29:u8[])
            n458 = Greater Than 0?(x=w44) -> (x > 0?=w43:bool)
          }
          frame 1, Default {
            n459 = Delete From Array(array=w56, length=14 ("index"), index=0 ("length")) -> (deleted portion=w49:u8[], array with subset deleted=w60:u8[])
            n460 = Array Size(array=w56) -> (size(s)=w55:i32)
            n461 = Array Size(array=w60) -> (size(s)=w59:i32)
            n462 = Replace Array Subset(array=w50, new element=w49, index=1) -> (w52:u8[])
            n463 = Greater?(x=w55, y=13 ("index")) -> (0:w54:bool)
            n464 = Greater Than 0?(x=w59) -> (x > 0?=w57:bool)
            n465 = Or(x=w54, y=w57) -> (x .or. y?=w58:bool)
          }
        }
      }
      n466 = Transpose 2D Array(2D array=w12) -> (transposed array=→"Downlink":u8[][])
    }
    frame Error {
    }
  }
  "error out" <- w2
